vi "Main - E700 Example.vi"() -> ()   [LabVIEW 2020]
uses:
  <vilib>/NI/Modbus Library/API/Master/Modbus Master.lvclass
  C:/Program Files (x86)/National Instruments/LabVIEW 2020/vi.lib/NI/Modbus Library/API/Modbus API.lvclass
  <vilib>/NI/Modbus Library/API/Modbus API.lvclass/Modbus API.ctl
  <vilib>/NI/Modbus Library/Transmission Data Unit/Transmission Data Unit.lvclass/Transmission Data Unit.ctl
  <vilib>/NI/Modbus Library/Transmission Data Unit/Write Unit ID.vi
  <vilib>/NI/Modbus Library/API/Read Transmission Data Unit.vi
  <vilib>/NI/Modbus Library/API/Write Transmission Data Unit.vi
  <vilib>/NI/Modbus Library/API/Wrapper/Create Serial Master.vi
  <vilib>/NI/Modbus Library/API/Wrapper/API Main.lvlib
panel:
  in  "Manual Vert Control 2":bool
  in  "Vertical Direction Switch 2":bool caption="Vertical Direction Switch"
  in  "Vertical Frequencey Setting (Hz) - Manual 2":dbl caption="Vertical Frequencey Setting (Hz)" min=0.0 max=60.0 step=1.0
  in  "Rotational Frequencey Setting (Hz) - Manual 2":dbl caption="Rotational Frequencey Setting (Hz)" min=0.0 max=60.0 step=1.0
  out "Tension":bool
  out "Grease":bool
  out "D-Shape":bool
  in  "Reset Tension":bool
  in  "Reset Grease":bool
  in  "Reset D Shape":bool
  in  "Full Automated Sequence":bool
  in  "Run Full Automated Sequence":string="Sequence 3\nSequence 4\nSequence 5\nSequence 6\nSequence 7\nSequence 8\nSequence 9\nSequence 10\nSequence 11\nSequence 12"
  out "Status":string
  in  "Manual Rotational Control":bool
  in  "Rotational Frequencey Setting (Hz) - Manual 1":dbl caption="Rotational Frequencey Setting (Hz)" min=0.0 max=60.0 step=1.0
  in  "Manual Vert Control":bool
  in  "Vertical Direction Switch":bool
  in  "Vertical Frequencey Setting (Hz) - Manual 1":dbl caption="Vertical Frequencey Setting (Hz)" min=0.0 max=60.0 step=1.0
  in  "Tab Control":T1(tab)
  in  "Seq 5 Direction Switch":bool
  in  "Seq5":bool
  in  "Time (mS) - Seq 5":u32=11400 caption="Time (mS)" max=60 step=1
  in  "Rotational Frequencey Setting (Hz) - Seq 5":dbl=9.4 caption="Rotational Frequencey Setting (Hz)" min=0.0 max=60.0 step=1.0
  in  "Vertical Frequencey Setting (Hz) - Seq 5":dbl caption="Vertical Frequencey Setting (Hz)" min=0.0 max=60.0 step=1.0
  in  "Seq 4 Direction Switch":bool
  in  "Seq4":bool
  in  "Time (mS) - Seq 4":u32=5600 caption="Time (mS)" max=60 step=1
  in  "Rotational Frequencey Setting (Hz) - Seq 4":dbl caption="Rotational Frequencey Setting (Hz)" min=0.0 max=60.0 step=1.0
  in  "Vertical Frequencey Setting (Hz) - Seq 4":dbl=30.0 caption="Vertical Frequencey Setting (Hz)" min=0.0 max=60.0 step=1.0
  in  "Seq 3 Direction Switch":bool
  in  "Seq3":bool
  in  "Time (mS) - Seq 3":u32=45050 caption="Time (mS)" max=60 step=1
  in  "Rotational Frequencey Setting (Hz) - Seq 3":dbl=9.4 caption="Rotational Frequencey Setting (Hz)" min=0.0 max=60.0 step=1.0
  in  "Vertical Frequencey Setting (Hz) - Seq 3":dbl=6.9 caption="Vertical Frequencey Setting (Hz)" min=0.0 max=60.0 step=1.0
  in  "Seq 2 Direction Switch":bool
  in  "Seq2":bool
  in  "Time (mS) - Seq 2":u32=6500 caption="Time (mS)" max=60 step=1
  in  "Rotational Frequencey Setting (Hz) - Seq 2":dbl=9.4 caption="Rotational Frequencey Setting (Hz)" min=0.0 max=60.0 step=1.0
  in  "Vertical Frequencey Setting (Hz) - Seq 2":dbl=6.9 caption="Vertical Frequencey Setting (Hz)" min=0.0 max=60.0 step=1.0
  in  "COM Port":refnum<visa-resource-name>
  in  "Seq 0 Direction Switch":bool
  in  "Seq0":bool
  in  "Time (mS) - Seq 0":u32=1500 caption="Time (mS)" max=60 step=1
  in  "Rotational Frequencey Setting (Hz) - Seq 0":dbl=9.4 caption="Rotational Frequencey Setting (Hz)" min=0.0 max=60.0 step=1.0
  in  "Vertical Frequencey Setting (Hz) - Seq 0":dbl caption="Vertical Frequencey Setting (Hz)" min=0.0 max=60.0 step=1.0
  in  "Seq 1 Direction Switch":bool
  in  "Seq1":bool
  in  "Time (mS) - Seq 1":u32=4000 caption="Time (mS)" max=60 step=1
  in  "Rotational Frequencey Setting (Hz) - Seq 1":dbl=9.4 caption="Rotational Frequencey Setting (Hz)" min=0.0 max=60.0 step=1.0
  in  "Vertical Frequencey Setting (Hz) - Seq 1":dbl=6.9 caption="Vertical Frequencey Setting (Hz)" min=0.0 max=60.0 step=1.0
  in  "Seq 6 Direction Switch":bool
  in  "Seq6":bool
  in  "Time (mS) - Seq 6":u32=60040 caption="Time (mS)" max=60 step=1
  in  "Rotational Frequencey Setting (Hz) - Seq 6":dbl=9.4 caption="Rotational Frequencey Setting (Hz)" min=0.0 max=60.0 step=1.0
  in  "Vertical Frequencey Setting (Hz) - Seq 6":dbl=5.4 caption="Vertical Frequencey Setting (Hz)" min=0.0 max=60.0 step=1.0
  in  "Seq 11 Direction Switch":bool
  in  "Seq11":bool
  in  "Time (mS) - Seq 11":u32=7600 caption="Time (mS)" max=60 step=1
  in  "Rotational Frequencey Setting (Hz) - Seq 11":dbl caption="Rotational Frequencey Setting (Hz)" min=0.0 max=60.0 step=1.0
  in  "Vertical Frequencey Setting (Hz) - Seq 11":dbl=30.0 caption="Vertical Frequencey Setting (Hz)" min=0.0 max=60.0 step=1.0
  in  "Seq 10 Direction Switch":bool
  in  "Seq10":bool
  in  "Time (mS) - Seq 10":u32=134850 caption="Time (mS)" max=60 step=1
  in  "Rotational Frequencey Setting (Hz) - Seq 10":dbl=9.4 caption="Rotational Frequencey Setting (Hz)" min=0.0 max=60.0 step=1.0
  in  "Vertical Frequencey Setting (Hz) - Seq 10":dbl=2.75 caption="Vertical Frequencey Setting (Hz)" min=0.0 max=60.0 step=1.0
  in  "Seq 9 Direction Switch":bool
  in  "Seq9":bool
  in  "Time (mS) - Seq 9":u32=45050 caption="Time (mS)" max=60 step=1
  in  "Rotational Frequencey Setting (Hz) - Seq 9":dbl=9.4 caption="Rotational Frequencey Setting (Hz)" min=0.0 max=60.0 step=1.0
  in  "Vertical Frequencey Setting (Hz) - Seq 9":dbl=5.4 caption="Vertical Frequencey Setting (Hz)" min=0.0 max=60.0 step=1.0
  in  "Seq 8 Direction Switch":bool
  in  "Seq8":bool
  in  "Time (mS) - Seq 8":u32=11400 caption="Time (mS)" max=60 step=1
  in  "Rotational Frequencey Setting (Hz) - Seq 8":dbl=9.4 caption="Rotational Frequencey Setting (Hz)" min=0.0 max=60.0 step=1.0
  in  "Vertical Frequencey Setting (Hz) - Seq 8":dbl caption="Vertical Frequencey Setting (Hz)" min=0.0 max=60.0 step=1.0
  in  "Seq 7 Direction Switch":bool
  in  "Seq7":bool
  in  "Time (mS) - Seq 7":u32=10900 caption="Time (mS)" max=60 step=1
  in  "Rotational Frequencey Setting (Hz) - Seq 7":dbl caption="Rotational Frequencey Setting (Hz)" min=0.0 max=60.0 step=1.0
  in  "Vertical Frequencey Setting (Hz) - Seq 7":dbl=30.0 caption="Vertical Frequencey Setting (Hz)" min=0.0 max=60.0 step=1.0
  in  "Seq 12 Direction Switch":bool
  in  "Seq12":bool
  in  "Time (mS) - Seq 12":u32=17034 caption="Time (mS)" max=60 step=1
  in  "Rotational Frequencey Setting (Hz) - Seq 12":dbl=9.4 caption="Rotational Frequencey Setting (Hz)" min=0.0 max=60.0 step=1.0
  in  "Vertical Frequencey Setting (Hz) - Seq 12":dbl=4.6 caption="Vertical Frequencey Setting (Hz)" min=0.0 max=60.0 step=1.0
  in  "Seq 15 Direction Switch":bool
  in  "Seq15":bool
  in  "Time (mS) - Seq 15":u32=13000 caption="Time (mS)" max=60 step=1
  in  "Rotational Frequencey Setting (Hz) - Seq 15":dbl=9.4 caption="Rotational Frequencey Setting (Hz)" min=0.0 max=60.0 step=1.0
  in  "Vertical Frequencey Setting (Hz) - Seq 15":dbl=4.6 caption="Vertical Frequencey Setting (Hz)" min=0.0 max=60.0 step=1.0
  in  "Seq 14 Direction Switch":bool
  in  "Seq14":bool
  in  "Time (mS) - Seq 14":u32=11060 caption="Time (mS)" max=60 step=1
  in  "Rotational Frequencey Setting (Hz) - Seq 14":dbl=9.4 caption="Rotational Frequencey Setting (Hz)" min=0.0 max=60.0 step=1.0
  in  "Vertical Frequencey Setting (Hz) - Seq 14":dbl=4.6 caption="Vertical Frequencey Setting (Hz)" min=0.0 max=60.0 step=1.0
  in  "Seq 13 Direction Switch":bool
  in  "Seq13":bool
  in  "Time (mS) - Seq 13":u32=4209 caption="Time (mS)" max=60 step=1
  in  "Rotational Frequencey Setting (Hz) - Seq 13":dbl=9.4 caption="Rotational Frequencey Setting (Hz)" min=0.0 max=60.0 step=1.0
  in  "Vertical Frequencey Setting (Hz) - Seq 13":dbl=4.6 caption="Vertical Frequencey Setting (Hz)" min=0.0 max=60.0 step=1.0
  out "Rotational Frequency Output":dbl
  out "Vertical Frequency Output":dbl
  in  "OK":bool
  # "Manual Control - Rotational"
  # "Manual Control-Vertical"
  # "Combination Control-Rotational and Vertical"
  # "Sequence 2 - Install Clamp at END and Turn Tension ON at END"
  # "Sequence 3 - Three Revolutions"
  # "Sequence 4 - Vertical Drop"
  # "Sequence 5 - 3/4 Turn Offset"
  # "Sequence 6 - Four Revolutions"
  # "Sequence 0 - Tension Offset and Start D at END"
  # "Sequence 1 - Start Grease at END"
  # "Sequence 7 - Vertical Drop"
  # "Sequence 8 - 3/4 Turn Offset"
  # "Sequence 9 - Three Revolutions"
  # "Sequence 10 - Nine Revolutions"
  # "Sequence 11 - Vertical Drop"
  # "Sequence 12 - One Revolution + 45 Degrees - Turn D off at END"
  # "Sequence 13 - 100 Degree Revolution, Turn Grease off at END"
  # "Sequence 14 - Finish Revolution and Install Clamp and Turn Tension OFF at END"
  # "Sequence 15 - Create Tail"
  # "Channel 79 needs to be set from 3 to 2 - Power must be cycled."
  # "21.5\" Diameter Tank:\nSequence 0 (mS): 1500\nSequence 1 (mS): 4000\nSequence 2 (mS): 6500\nSequence 3 (mS): 45000\nSequence 4 (mS): 5600\nSequence 5 (mS): 11500\nSequence 6 (mS): 50000\nSequence 7 (mS): 10900\nSequence 8 (mS): 10500\nSequence 9 (mS): 33750\nSequence 10 (mS): 137000\nSequence 11 (mS): 7600\nSequence 12 (mS): 16500\nSequence 13 (mS): 3000 \nSequence 14 (mS): 10000\nSequence 15 (mS): 13000"
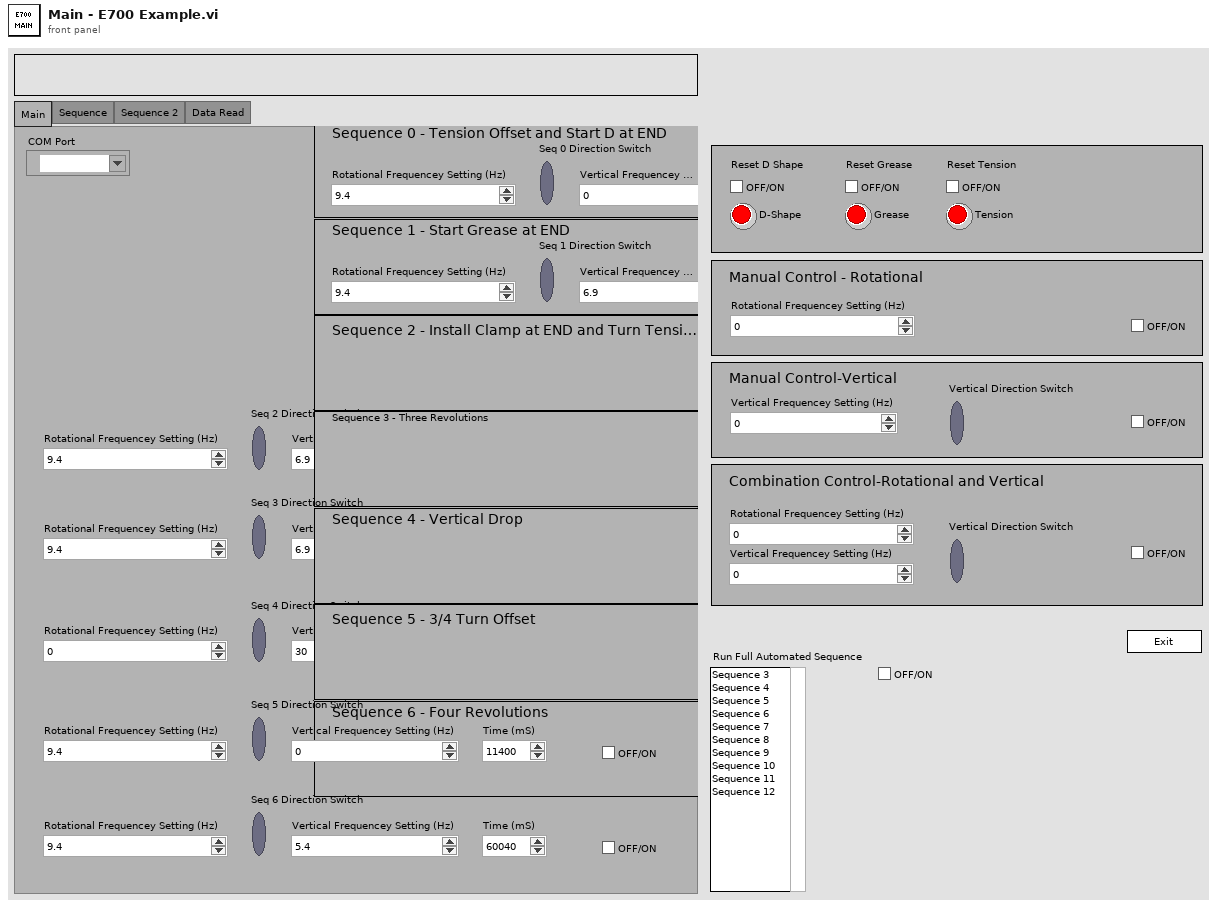
[diagram p1: front panel]
types:
  T1 = enum32{"Main", "Sequence", "Sequence 2", "Data Read"}
  T2 = enum32{"Invalid", "Standard", "Closed", "Hidden", "Minimized", "Maximized"}
  T3 = enum32{"invalid app kind", "Development System", "Run Time System", "Student Edition", "Embedded LabVIEW", "Evaluation", "Custom"}
  T4 = cluster{"Core":cluster{"Current VI Reference":refnum<vi>, "Close Panel on Exit?":bool}, "COM Port":refnum<visa-resource-name>, "Rotation Instance":refnum<class "Modbus Master.lvclass">, "Tension":bool, "D Shape":bool, "Grease":bool}
  T5 = cluster{"Current VI Reference":refnum<vi>, "Close Panel on Exit?":bool}
  T6 = cluster{"register values[0]":u16, "register values[1]":u16, "register values[2]":u16, "register values[3]":u16, "register values[4]":u16, "register values[5]":u16, "register values[6]":u16, "register values[7]":u16, "register values[8]":u16}
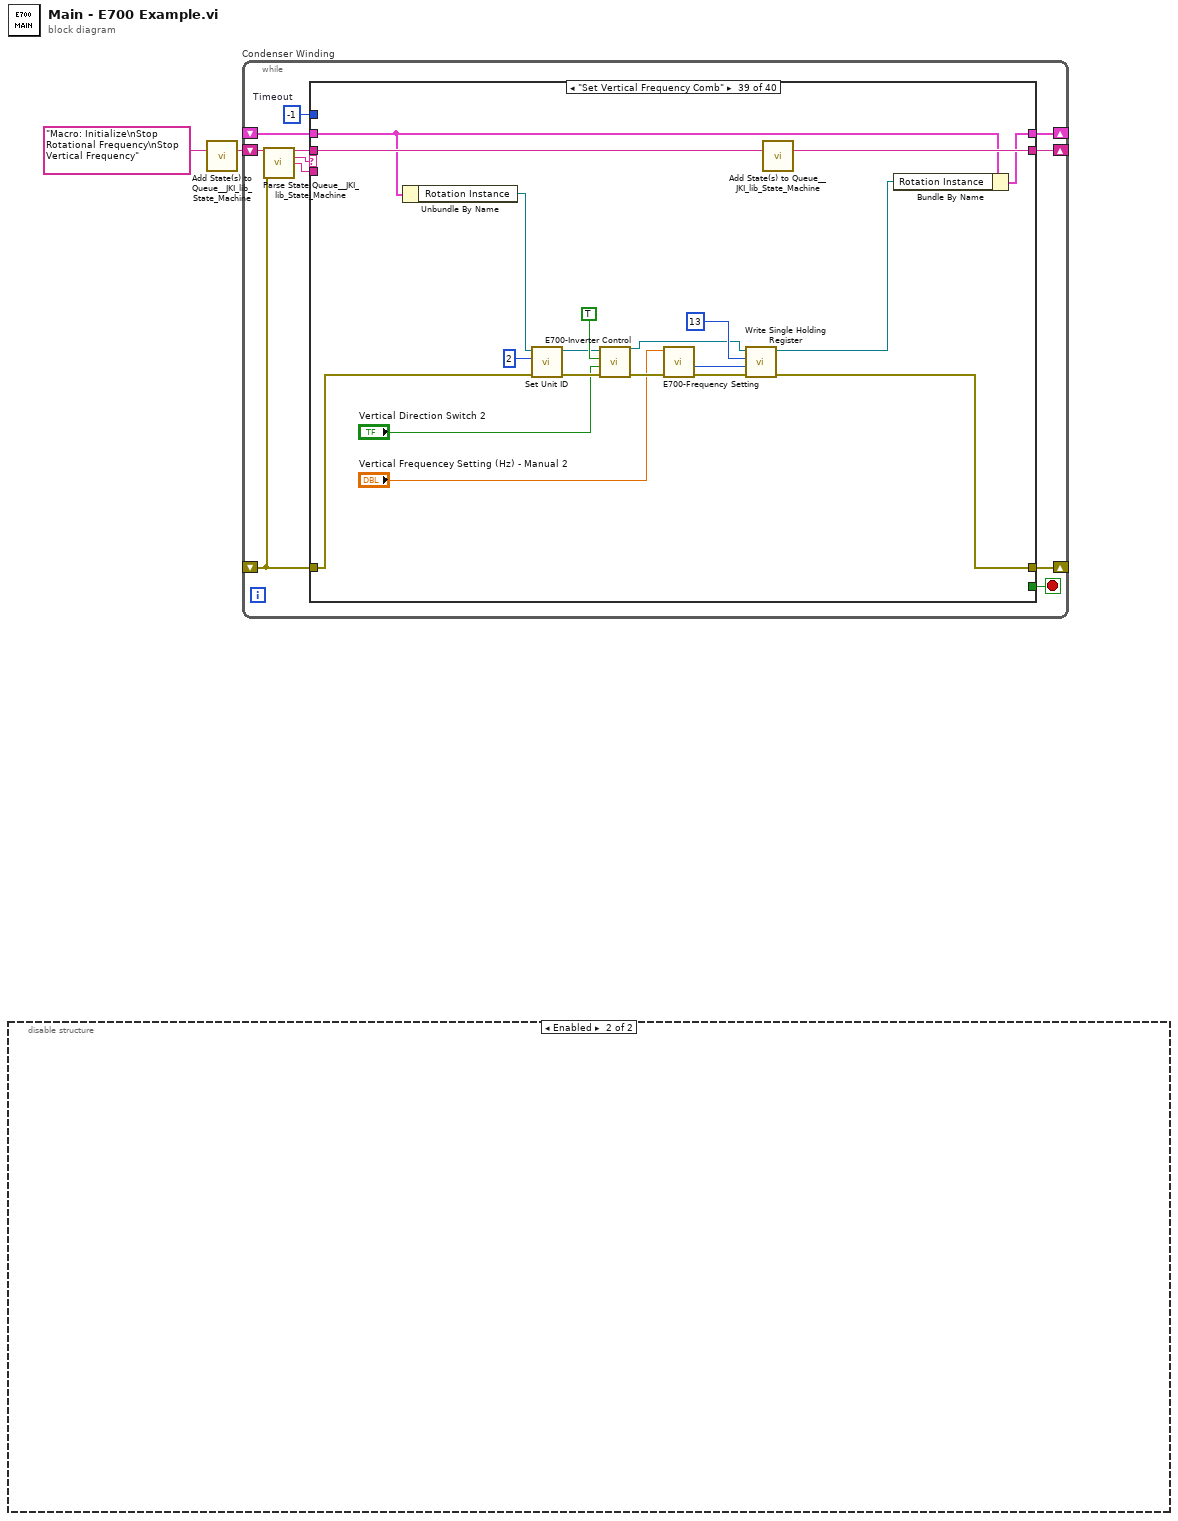
[diagram p0: block diagram]
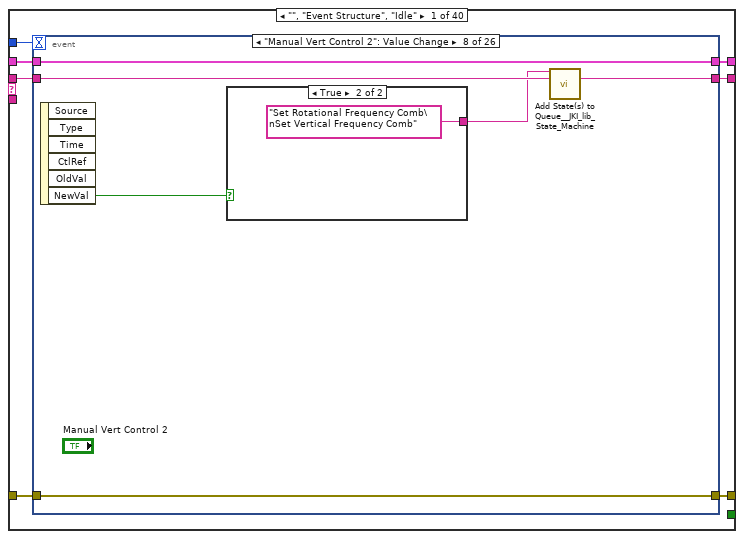
[diagram p2: hidden frame]
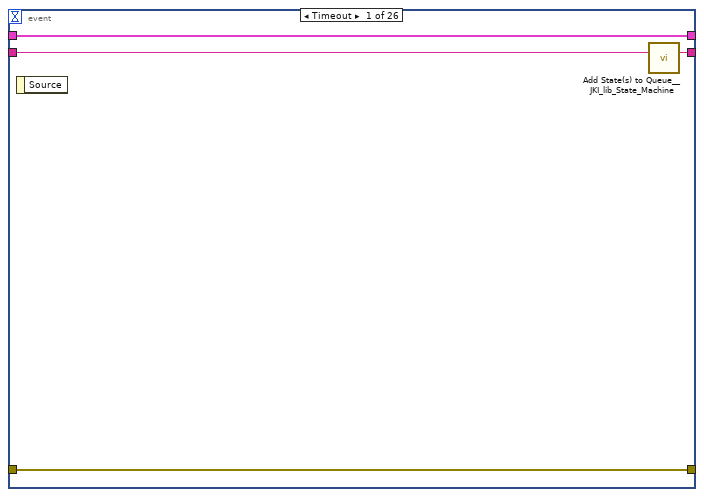
[diagram p3: hidden frame]
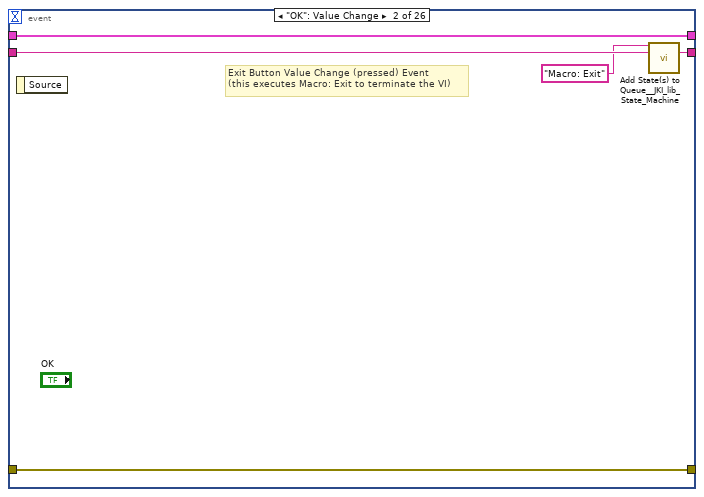
[diagram p4: hidden frame]
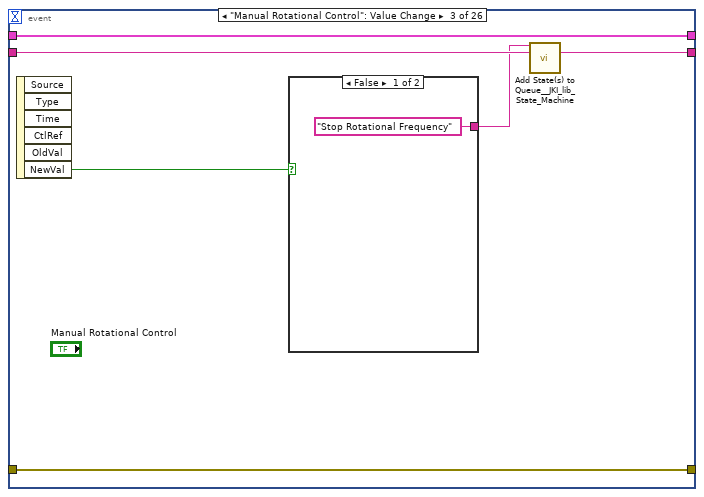
[diagram p5: hidden frame]
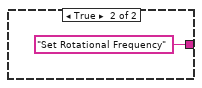
[diagram p6: hidden frame]
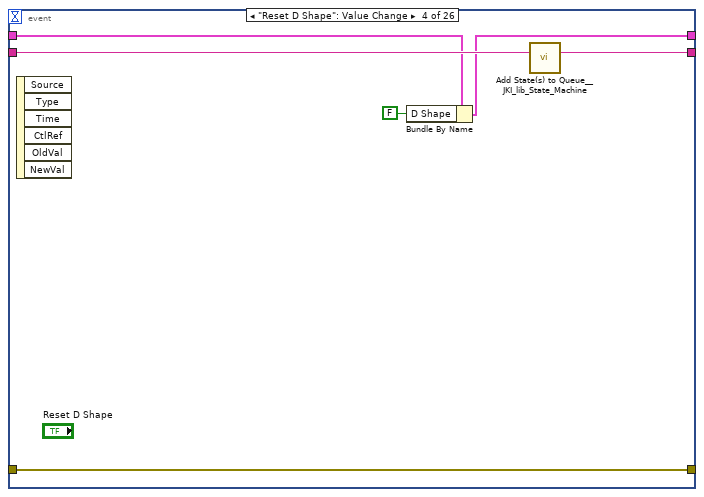
[diagram p7: hidden frame]
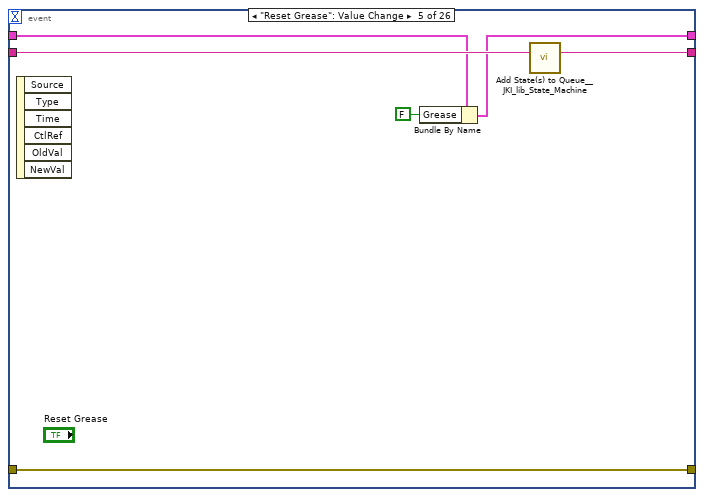
[diagram p8: hidden frame]
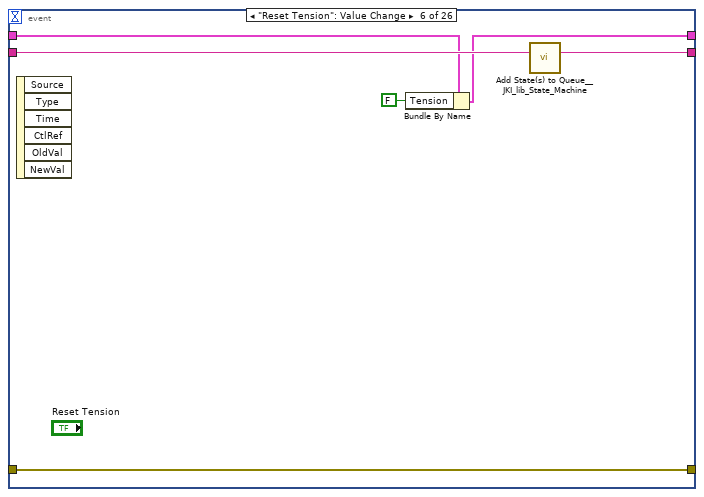
[diagram p9: hidden frame]
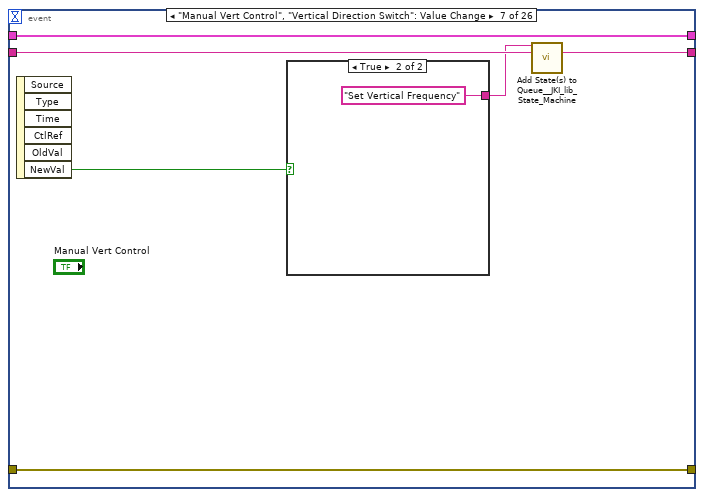
[diagram p10: hidden frame]
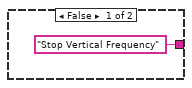
[diagram p11: hidden frame]
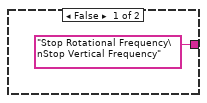
[diagram p12: hidden frame]
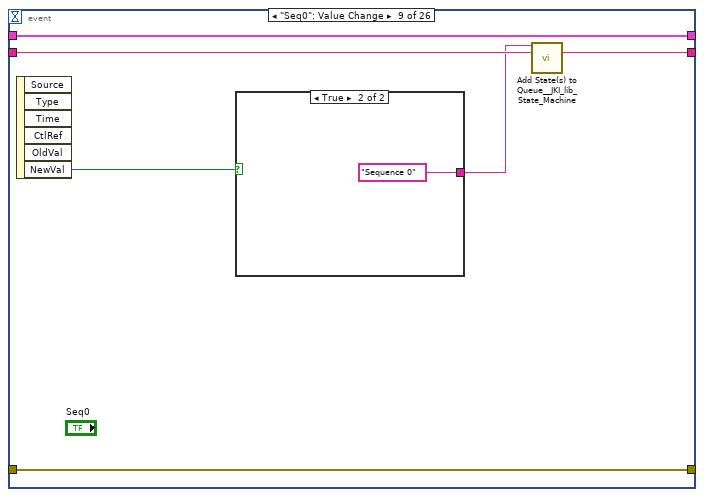
[diagram p13: hidden frame]
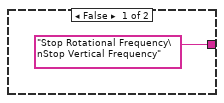
[diagram p14: hidden frame]
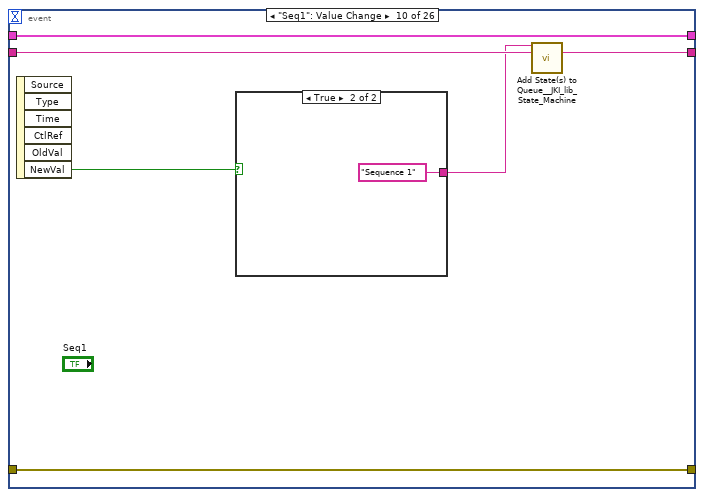
[diagram p15: hidden frame]
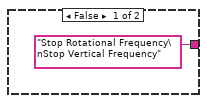
[diagram p16: hidden frame]
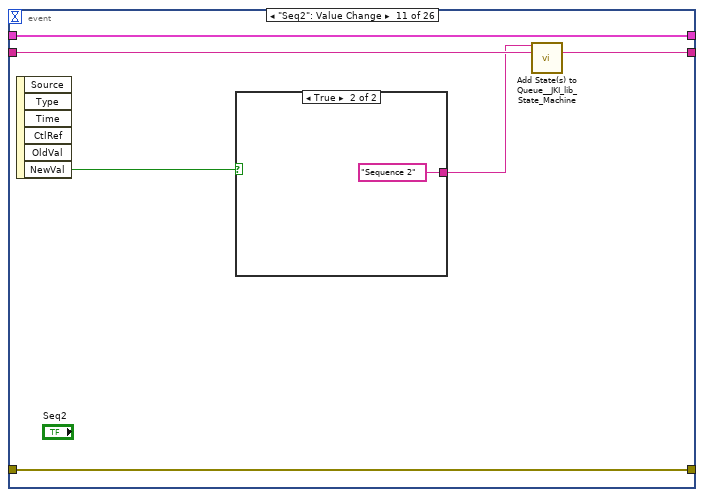
[diagram p17: hidden frame]
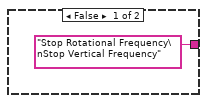
[diagram p18: hidden frame]
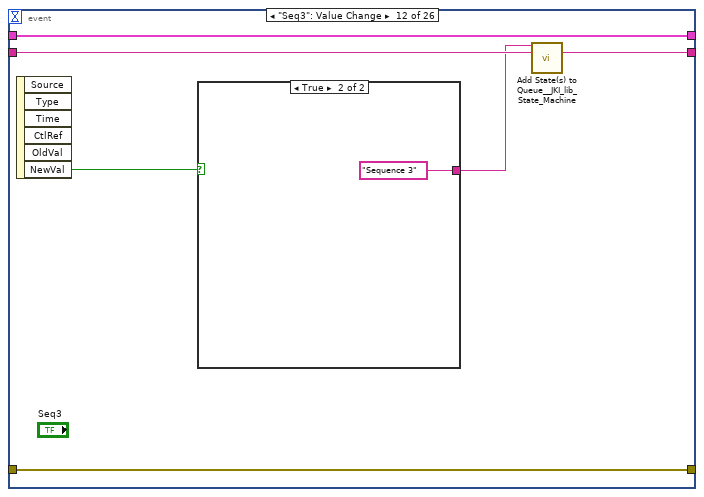
[diagram p19: hidden frame]
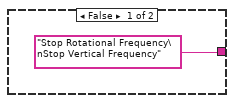
[diagram p20: hidden frame]
diagram:
  n1 = disable-structure shown="Enabled" {
    frame Disabled {
    }
    frame Enabled {
    }
  }
  n2 = call <vilib>:"Add State(s) to Queue__JKI_lib_State_Machine.vi"("State(s) in (\"\")"="Macro: Initialize\nStop Rotational Frequency\nStop Vertical Frequency") -> ("States Out"=w2:string)  [unwired: 14 in]
  n3 = while "Condenser Winding" {
    shift-right: [w6] -> _
    shift-left: _ -> [w5]
    shift-right: [w9] -> _
    shift-left: _ -> [w3]
    shift-right: [w8] -> _
    shift-left: w2 -> [w10]
    stop <- w7 stop-if-true
    w4 = -1  # Timeout
    n4 = call <vilib>:"Parse State Queue__JKI_lib_State_Machine.vi"("State Queue"=w10, "Error In (no error)"=w3) -> ("Remaining States"=w12:string, "Current State"=w13:string, "Arguments"=w11:string)  [unwired: 11 in]
    n5 = case shown="\"Set Vertical Frequency Comb\"" w13 {
      selector: w13 -> [_ _ w218 _ _ _ _ _ _ _ _ _ _ _ _ _ _ _ _ _ _ _ _ _ _ _ _ _ _ _ _ _ _ _ _ _ _ _ _ _]
      tunnel: w12 -> [w20 w217 w222 w241 w247 w254 w258 w268 w274 w278 w292 w298 w309 w378 w383 w393 w397 w410 w427 w444 w459 w472 w489 w504 w517 w534 w549 w560 w573 w592 w613 w630 w645 w650 w687 w702 w717 w736 w755 w767]
      tunnel: w11 -> [_ _ _ _ _ _ _ _ _ _ _ w293 w303 _ _ _ _ _ _ _ _ _ _ _ _ _ _ _ _ _ _ _ _ _ _ _ _ _ _ _]
      tunnel: w5 -> [w18 w214 w220 w234 w244 w251 w255 _ w269 w275 w284 w296 w305 w375 w380 w390 w394 w399 w415 w432 w457 w464 w481 w502 w509 w526 w547 w558 w565 w581 w603 w619 w643 w648 w681 w696 w711 w730 w749 w764]
      tunnel: [w17 w215 w224 w238 errorcluster {"status"=FALSE, "code"=0, "source"=""} ("error out") w250 w256 w265 w270 w276 w280 w294 w306 w376 w381 w391 w395 w400 w417 w434 w455 w461 w477 w496 w505 w522 w544 w555 w561 w583 w601 w618 w640 w646 w682 w697 w712 w718 w739 w763] -> w9
      tunnel: w3 -> [w16 w215 w223 w238 w243 w248 w256 w265 w271 w276 w286 w295 w307 w376 w381 w391 w395 w408 w425 w441 w456 w463 w479 w501 w507 w523 w546 w557 w563 w579 w611 w628 w642 w647 w683 w698 w713 w722 w743 w757]
      tunnel: [w19 w216 w221 w240 w246 w253 w257 w267 w273 w277 w291 w297 w308 w377 w382 w392 w396 w409 w426 w443 w458 w471 w488 w503 w516 w533 w548 w559 w572 w591 w612 w629 w644 w649 w686 w701 w716 w735 w754 w766] -> w8
      tunnel: [_ _ _ _ _ TRUE _ _ _ _ _ _ _ _ _ _ _ _ _ _ _ _ _ _ _ _ _ _ _ _ _ _ _ _ _ _ _ _ _ _] -> w7
      tunnel: [w15 w214 w220 w239 w244 w251 w255 w266 w269 w275 w283 w296 w305 w375 w380 w390 w394 w398 w416 w433 w457 w460 w478 w502 w508 w525 w547 w558 w564 w582 w604 w620 w643 w648 w680 w695 w710 w731 w750 w765] -> w6
      tunnel: w4 -> [w14 _ _ _ _ _ _ _ _ _ _ _ _ _ _ _ _ _ _ _ _ _ _ _ _ _ _ _ _ _ _ _ _ _ _ _ _ _ _ _]
      frame "", "Event Structure", "Idle" {
        n6 = event shown="[7] \"Manual Vert Control 2\": Value Change" {
          selector: _ -> [_ _ _ _ _ _ _ _ _ _ _ _ _ _ _ _ _ _ _ _ _ _ _ _ _ _]
          dyn-events: _ -> [_ _ _ _ _ _ _ _ _ _ _ _ _ _ _ _ _ _ _ _ _ _ _ _ _ _]
          timeout: w14 -> [_ _ _ _ _ _ _ _ _ _ _ _ _ _ _ _ _ _ _ _ _ _ _ _ _ _]
          tunnel: w20 -> [w24 w29 w34 w43 w49 w55 w58 w67 w74 w82 w90 w98 w106 w114 w122 w130 w138 w146 w154 w162 w170 w178 w186 w194 w202 w213]
          tunnel: [w23 w28 w33 w42 w48 w54 w59 w66 w75 w83 w91 w99 w107 w115 w123 w131 w139 w147 w155 w163 w171 w179 w187 w195 w203 w212] -> w19
          tunnel: w18 -> [w21 w26 w35 w40 w46 w52 w61 w69 w77 w85 w93 w101 w109 w117 w125 w133 w141 w149 w157 w165 w173 w181 w189 w197 w205 w210]
          tunnel: [w22 w27 w31 w41 w47 w53 w60 w68 w76 w84 w92 w100 w108 w116 w124 w132 w140 w148 w156 w164 w172 w180 w188 w196 w204 w211] -> w17
          tunnel: w16 -> [w22 w27 w31 w41 w47 w53 w60 w68 w76 w84 w92 w100 w108 w116 w124 w132 w140 w148 w156 w164 w172 w180 w188 w196 w204 w211]
          tunnel: [w21 w26 w35 w39 w45 w51 w61 w69 w77 w85 w93 w101 w109 w117 w125 w133 w141 w149 w157 w165 w173 w181 w189 w197 w205 w210] -> w15
          event Timeout {
            n7 = event-data() -> ()  [unwired: 1 in, 1 out]
            n8 = call <vilib>:"Add State(s) to Queue__JKI_lib_State_Machine.vi"("State(s) in (\"\")"=w24) -> ("States Out"=w23:string)  [unwired: 14 in]
          }
          event "OK": Value Change {
            # "Exit Button Value Change (pressed) Event\n(this executes Macro: Exit to terminate the VI)"
            n9 = event-data() -> ()  [unwired: 1 in, 1 out]
            n10 = call <vilib>:"Add State(s) to Queue__JKI_lib_State_Machine.vi"("State(s) in Front (\"\")"="Macro: Exit", "State(s) in (\"\")"=w29) -> ("States Out"=w28:string)  [unwired: 13 in]
          }
          event "Manual Rotational Control": Value Change {
            n11 = event-data() -> ("NewVal"=w30:bool)  [unwired: 1 in, 5 out]
            n12 = case shown="False" w30 {
              tunnel: ["Stop Rotational Frequency" ("State(s) in Front (\"\")") "Set Rotational Frequency" ("State(s) in Front (\"\")")] -> w32
              frame False {
              }
              frame True {
              }
            }
            n13 = call <vilib>:"Add State(s) to Queue__JKI_lib_State_Machine.vi"("State(s) in Front (\"\")"=w32, "State(s) in (\"\")"=w34) -> ("States Out"=w33:string)  [unwired: 13 in]
          }
          event "Reset D Shape": Value Change {
            n14 = event-data() -> ()  [unwired: 1 in, 6 out]
            n15 = Bundle By Name(cluster=w40, "D Shape"=FALSE) -> (w39:T4)
            n16 = call <vilib>:"Add State(s) to Queue__JKI_lib_State_Machine.vi"("State(s) in (\"\")"=w43) -> ("States Out"=w42:string)  [unwired: 14 in]
          }
          event "Reset Grease": Value Change {
            n17 = event-data() -> ()  [unwired: 1 in, 6 out]
            n18 = Bundle By Name(cluster=w46, "Grease"=FALSE) -> (w45:T4)
            n19 = call <vilib>:"Add State(s) to Queue__JKI_lib_State_Machine.vi"("State(s) in (\"\")"=w49) -> ("States Out"=w48:string)  [unwired: 14 in]
          }
          event "Reset Tension": Value Change {
            n20 = event-data() -> ()  [unwired: 1 in, 6 out]
            n21 = Bundle By Name(cluster=w52, "Tension"=FALSE) -> (w51:T4)
            n22 = call <vilib>:"Add State(s) to Queue__JKI_lib_State_Machine.vi"("State(s) in (\"\")"=w55) -> ("States Out"=w54:string)  [unwired: 14 in]
          }
          event "Manual Vert Control", "Vertical Direction Switch": Value Change {
            n23 = event-data() -> ("NewVal"=w56:bool)  [unwired: 1 in, 5 out]
            n24 = case shown="True" w56 {
              tunnel: ["Stop Vertical Frequency" ("State(s) in Front (\"\")") "Set Vertical Frequency" ("State(s) in Front (\"\")")] -> w57
              frame False {
              }
              frame True {
              }
            }
            n25 = call <vilib>:"Add State(s) to Queue__JKI_lib_State_Machine.vi"("State(s) in Front (\"\")"=w57, "State(s) in (\"\")"=w58) -> ("States Out"=w59:string)  [unwired: 13 in]
          }
          event "Manual Vert Control 2": Value Change {
            n26 = event-data() -> ("NewVal"=w65:bool)  [unwired: 1 in, 5 out]
            n27 = case shown="True" w65 {
              tunnel: ["Stop Rotational Frequency\nStop Vertical Frequency" ("State(s) in Front (\"\")") "Set Rotational Frequency Comb\nSet Vertical Frequency Comb" ("State(s) in Front (\"\")")] -> w64
              frame False {
              }
              frame True {
              }
            }
            n28 = call <vilib>:"Add State(s) to Queue__JKI_lib_State_Machine.vi"("State(s) in Front (\"\")"=w64, "State(s) in (\"\")"=w67) -> ("States Out"=w66:string)  [unwired: 13 in]
          }
          event "Seq0": Value Change {
            n29 = event-data() -> ("NewVal"=w72:bool)  [unwired: 1 in, 5 out]
            n30 = case shown="True" w72 {
              tunnel: ["Stop Rotational Frequency\nStop Vertical Frequency" ("State(s) in Front (\"\")") "Sequence 0" ("State(s) in Front (\"\")")] -> w73
              frame False {
              }
              frame True {
              }
            }
            n31 = call <vilib>:"Add State(s) to Queue__JKI_lib_State_Machine.vi"("State(s) in Front (\"\")"=w73, "State(s) in (\"\")"=w74) -> ("States Out"=w75:string)  [unwired: 13 in]
          }
          event "Seq1": Value Change {
            n32 = event-data() -> ("NewVal"=w80:bool)  [unwired: 1 in, 5 out]
            n33 = case shown="True" w80 {
              tunnel: ["Stop Rotational Frequency\nStop Vertical Frequency" ("State(s) in Front (\"\")") "Sequence 1" ("State(s) in Front (\"\")")] -> w81
              frame False {
              }
              frame True {
              }
            }
            n34 = call <vilib>:"Add State(s) to Queue__JKI_lib_State_Machine.vi"("State(s) in Front (\"\")"=w81, "State(s) in (\"\")"=w82) -> ("States Out"=w83:string)  [unwired: 13 in]
          }
          event "Seq2": Value Change {
            n35 = event-data() -> ("NewVal"=w88:bool)  [unwired: 1 in, 5 out]
            n36 = case shown="True" w88 {
              tunnel: ["Stop Rotational Frequency\nStop Vertical Frequency" ("State(s) in Front (\"\")") "Sequence 2" ("State(s) in Front (\"\")")] -> w89
              frame False {
              }
              frame True {
              }
            }
            n37 = call <vilib>:"Add State(s) to Queue__JKI_lib_State_Machine.vi"("State(s) in Front (\"\")"=w89, "State(s) in (\"\")"=w90) -> ("States Out"=w91:string)  [unwired: 13 in]
          }
          event "Seq3": Value Change {
            n38 = event-data() -> ("NewVal"=w96:bool)  [unwired: 1 in, 5 out]
            n39 = case shown="True" w96 {
              tunnel: ["Stop Rotational Frequency\nStop Vertical Frequency" ("State(s) in Front (\"\")") "Sequence 3" ("State(s) in Front (\"\")")] -> w97
              frame False {
              }
              frame True {
              }
            }
            n40 = call <vilib>:"Add State(s) to Queue__JKI_lib_State_Machine.vi"("State(s) in Front (\"\")"=w97, "State(s) in (\"\")"=w98) -> ("States Out"=w99:string)  [unwired: 13 in]
          }
          event "Seq4": Value Change {
            n41 = event-data() -> ("NewVal"=w104:bool)  [unwired: 1 in, 5 out]
            n42 = case shown="True" w104 {
              tunnel: ["Stop Rotational Frequency\nStop Vertical Frequency" ("State(s) in Front (\"\")") "Sequence 4" ("State(s) in Front (\"\")")] -> w105
              frame False {
              }
              frame True {
              }
            }
            n43 = call <vilib>:"Add State(s) to Queue__JKI_lib_State_Machine.vi"("State(s) in Front (\"\")"=w105, "State(s) in (\"\")"=w106) -> ("States Out"=w107:string)  [unwired: 13 in]
          }
          event "Seq5": Value Change {
            n44 = event-data() -> ("NewVal"=w112:bool)  [unwired: 1 in, 5 out]
            n45 = case shown="True" w112 {
              tunnel: ["Stop Rotational Frequency\nStop Vertical Frequency" ("State(s) in Front (\"\")") "Sequence 5" ("State(s) in Front (\"\")")] -> w113
              frame False {
              }
              frame True {
              }
            }
            n46 = call <vilib>:"Add State(s) to Queue__JKI_lib_State_Machine.vi"("State(s) in Front (\"\")"=w113, "State(s) in (\"\")"=w114) -> ("States Out"=w115:string)  [unwired: 13 in]
          }
          event "Seq6": Value Change {
            n47 = event-data() -> ("NewVal"=w120:bool)  [unwired: 1 in, 5 out]
            n48 = case shown="True" w120 {
              tunnel: ["Stop Rotational Frequency\nStop Vertical Frequency" ("State(s) in Front (\"\")") "Sequence 6" ("State(s) in Front (\"\")")] -> w121
              frame False {
              }
              frame True {
              }
            }
            n49 = call <vilib>:"Add State(s) to Queue__JKI_lib_State_Machine.vi"("State(s) in Front (\"\")"=w121, "State(s) in (\"\")"=w122) -> ("States Out"=w123:string)  [unwired: 13 in]
          }
          event "Seq7": Value Change {
            n50 = event-data() -> ("NewVal"=w128:bool)  [unwired: 1 in, 5 out]
            n51 = case shown="True" w128 {
              tunnel: ["Stop Rotational Frequency\nStop Vertical Frequency" ("State(s) in Front (\"\")") "Sequence 7" ("State(s) in Front (\"\")")] -> w129
              frame False {
              }
              frame True {
              }
            }
            n52 = call <vilib>:"Add State(s) to Queue__JKI_lib_State_Machine.vi"("State(s) in Front (\"\")"=w129, "State(s) in (\"\")"=w130) -> ("States Out"=w131:string)  [unwired: 13 in]
          }
          event "Seq8": Value Change {
            n53 = event-data() -> ("NewVal"=w136:bool)  [unwired: 1 in, 5 out]
            n54 = case shown="True" w136 {
              tunnel: ["Stop Rotational Frequency\nStop Vertical Frequency" ("State(s) in Front (\"\")") "Sequence 8" ("State(s) in Front (\"\")")] -> w137
              frame False {
              }
              frame True {
              }
            }
            n55 = call <vilib>:"Add State(s) to Queue__JKI_lib_State_Machine.vi"("State(s) in Front (\"\")"=w137, "State(s) in (\"\")"=w138) -> ("States Out"=w139:string)  [unwired: 13 in]
          }
          event "Seq9": Value Change {
            n56 = event-data() -> ("NewVal"=w144:bool)  [unwired: 1 in, 5 out]
            n57 = case shown="True" w144 {
              tunnel: ["Stop Rotational Frequency\nStop Vertical Frequency" ("State(s) in Front (\"\")") "Sequence 9" ("State(s) in Front (\"\")")] -> w145
              frame False {
              }
              frame True {
              }
            }
            n58 = call <vilib>:"Add State(s) to Queue__JKI_lib_State_Machine.vi"("State(s) in Front (\"\")"=w145, "State(s) in (\"\")"=w146) -> ("States Out"=w147:string)  [unwired: 13 in]
          }
          event "Seq10": Value Change {
            n59 = event-data() -> ("NewVal"=w152:bool)  [unwired: 1 in, 5 out]
            n60 = case shown="True" w152 {
              tunnel: ["Stop Rotational Frequency\nStop Vertical Frequency" ("State(s) in Front (\"\")") "Sequence 10" ("State(s) in Front (\"\")")] -> w153
              frame False {
              }
              frame True {
              }
            }
            n61 = call <vilib>:"Add State(s) to Queue__JKI_lib_State_Machine.vi"("State(s) in Front (\"\")"=w153, "State(s) in (\"\")"=w154) -> ("States Out"=w155:string)  [unwired: 13 in]
          }
          event "Seq11": Value Change {
            n62 = event-data() -> ("NewVal"=w160:bool)  [unwired: 1 in, 5 out]
            n63 = case shown="True" w160 {
              tunnel: ["Stop Rotational Frequency\nStop Vertical Frequency" ("State(s) in Front (\"\")") "Sequence 11" ("State(s) in Front (\"\")")] -> w161
              frame False {
              }
              frame True {
              }
            }
            n64 = call <vilib>:"Add State(s) to Queue__JKI_lib_State_Machine.vi"("State(s) in Front (\"\")"=w161, "State(s) in (\"\")"=w162) -> ("States Out"=w163:string)  [unwired: 13 in]
          }
          event "Seq12": Value Change {
            n65 = event-data() -> ("NewVal"=w168:bool)  [unwired: 1 in, 5 out]
            n66 = case shown="True" w168 {
              tunnel: ["Stop Rotational Frequency\nStop Vertical Frequency" ("State(s) in Front (\"\")") "Sequence 12" ("State(s) in Front (\"\")")] -> w169
              frame False {
              }
              frame True {
              }
            }
            n67 = call <vilib>:"Add State(s) to Queue__JKI_lib_State_Machine.vi"("State(s) in Front (\"\")"=w169, "State(s) in (\"\")"=w170) -> ("States Out"=w171:string)  [unwired: 13 in]
          }
          event "Seq13": Value Change {
            n68 = event-data() -> ("NewVal"=w176:bool)  [unwired: 1 in, 5 out]
            n69 = case shown="True" w176 {
              tunnel: ["Stop Rotational Frequency\nStop Vertical Frequency" ("State(s) in Front (\"\")") "Sequence 13" ("State(s) in Front (\"\")")] -> w177
              frame False {
              }
              frame True {
              }
            }
            n70 = call <vilib>:"Add State(s) to Queue__JKI_lib_State_Machine.vi"("State(s) in Front (\"\")"=w177, "State(s) in (\"\")"=w178) -> ("States Out"=w179:string)  [unwired: 13 in]
          }
          event "Seq14": Value Change {
            n71 = event-data() -> ("NewVal"=w184:bool)  [unwired: 1 in, 5 out]
            n72 = case shown="True" w184 {
              tunnel: ["Stop Rotational Frequency\nStop Vertical Frequency" ("State(s) in Front (\"\")") "Sequence 14" ("State(s) in Front (\"\")")] -> w185
              frame False {
              }
              frame True {
              }
            }
            n73 = call <vilib>:"Add State(s) to Queue__JKI_lib_State_Machine.vi"("State(s) in Front (\"\")"=w185, "State(s) in (\"\")"=w186) -> ("States Out"=w187:string)  [unwired: 13 in]
          }
          event "Seq15": Value Change {
            n74 = event-data() -> ("NewVal"=w192:bool)  [unwired: 1 in, 5 out]
            n75 = case shown="True" w192 {
              tunnel: ["Stop Rotational Frequency\nStop Vertical Frequency" ("State(s) in Front (\"\")") "Sequence 15" ("State(s) in Front (\"\")")] -> w193
              frame False {
              }
              frame True {
              }
            }
            n76 = call <vilib>:"Add State(s) to Queue__JKI_lib_State_Machine.vi"("State(s) in Front (\"\")"=w193, "State(s) in (\"\")"=w194) -> ("States Out"=w195:string)  [unwired: 13 in]
          }
          event "Full Automated Sequence": Value Change {
            n77 = event-data() -> ("NewVal"=w200:bool)  [unwired: 1 in, 5 out]
            n78 = case shown="False" w200 {
              tunnel: ["Stop Rotational Frequency\nStop Vertical Frequency" ("State(s) in Front (\"\")") "Run Full Automated Sequence"] -> w201
              frame False {
              }
              frame True {
              }
            }
            n79 = call <vilib>:"Add State(s) to Queue__JKI_lib_State_Machine.vi"("State(s) in Front (\"\")"=w201, "State(s) in (\"\")"=w202) -> ("States Out"=w203:string)  [unwired: 13 in]
          }
          event Panel Close? {
            # "Discard the event because we'll close the front panel ourselves in Macro: Exit"
            # "Close Panel button (pressed) Event\n(this executes Macro: Exit to terminate the VI)"
            n80 = event-data() -> ()  [unwired: 1 in, 1 out]
            n81 = event-data("Discard?"=TRUE) -> ()  [unwired: 1 in, 1 out]
            n82 = call <vilib>:"Add State(s) to Queue__JKI_lib_State_Machine.vi"("State(s) in Front (\"\")"="Macro: Exit", "State(s) in (\"\")"=w213) -> ("States Out"=w212:string)  [unwired: 13 in]
          }
        }
      }
      frame "---------- Core ----------" {
        # "Do not put any code in this frame.\n(it is a separator no-op)"
        n83 = call <vilib>:"Add State(s) to Queue__JKI_lib_State_Machine.vi"("State(s) in (\"\")"=w217) -> ("States Out"=w216:string)  [unwired: 14 in]
      }
      frame Default {
        w227 = 42 items=["No error", "Argument error", "Memory is full", "Out of zone", "End of file", "File already open", "Generic file I/O error", "File not found", "File permission error", "Disk is full", "Duplicate path", "Too many files open", "System feature not enabled", "Resource file not found", "Cannot add resource", "Resource not found", "Image not found", "Image memory error", "Pen does not exist", "Config type invalid", "Config token not found", "Config parse error", "Config memory error", "Bad external code format", "Bad external code offset", "External code not present", "Null window", "Destroy window error", "Null menu", "Print aborted", "Bad print record", "Print driver error", "Windows error during printing", "Memory error during printing", "Print dialog error", "Generic print error", "Invalid device refnum", "Device not found", "Device parameter error", "Device unit error", "Cannot open device", "Device call aborted", "Generic error", "Cancelled by user", "Object ID too low", "Object ID too high", "Object not in heap", "Unknown heap", "Unknown object (invalid DefProc)", "Unknown object (DefProc not in table)", "Message out of range", "Invalid (null) method", "Unknown message", "Manager call not supported", "Bad address", "Network operation in progress", "Network operation timed out", "Connection is busy", "Network attribute not supported", "Network error", "Address in use", "System out of memory", "Connection aborted", "Connection refused", "Not connected", "Already connected", "Connection closed", "Initialization error (interapplication manager)", "Bad occurrence", "Wait on unbound occurrence handler", "Occurrence queue overflow", "Datalog type conflict", "Unused", "Unrecognized type (interapplication manager)", "Memory corrupt", "Failed to make temporary DLL", "Old CIN version", "Drag socket not found", "Failed to load drop-object", "Failed to register OLE object", "Failed to release OLE object", "Format specifier type mismatch", "Unknown format specifier", "Too few format specifiers", "Too many format specifiers", "Scan failed", "Newer CIN version", "Error converting to variant", "Runtime menu error", "Password tampered", "Variant attribute not found", "Incompatible variant data type", "Event data is not available", "Event Store is not present", "Occurrence is not found", "Event Queue is not created", "Event info is not available", "Refnum passed is NULL", "Error retrieving Class GUID", "Error retrieving CoClass GUID", "Error retrieving TypeLib GUID.", "Bad built application magic bytes.", "Specific driver is different from the specific driver associated with the Logical Name.", "There is no session opened to the class driver.", "Max Error", "MAX - Error with config objects", "MAX - Error loading configuration", "MAX - Group not supported"]
        # "Current State"
        # "Do not delete, rename, or modify this frame.\n(this is used to capture unhandled states and typos)"
        # "Handle mistyped state name (developer tool)"
        n84 = Format Into String(format string="Software Exception: Unhandled State \"%s\"." ("message"), error in=w223, w218) -> (resulting string=w226:string, error out=w225:errorcluster)  [unwired: 1 in]
        n85 = call <vilib>:"Error Cluster From Error Code.vi"("show call chain? (False)"=TRUE, "error in (no error)"=w225, "error message (\"\")"=w226, "error code (0)"=w227) -> ("error out"=w224:errorcluster)  [unwired: 5 in]
        n86 = call <vilib>:"Add State(s) to Queue__JKI_lib_State_Machine.vi"("State(s) in (\"\")"=w222) -> ("States Out"=w221:string)  [unwired: 14 in]
      }
      frame "Initialize Core Data" {
        # "Do not delete, rename, or modify this frame.\n(this is used to determine panel behavior on exit)"
        # "originally closed?"
        # "exe?"
        # "If panel starts closed or is an EXE, then close it when we exit"
        n87 = property class="VI"() -> ("FP.State"=w231:T2)  [unwired: 2 in, 2 out]
        n88 = property class="App"() -> ("App.Kind"=w237:T3)  [unwired: 2 in, 2 out]
        n89 = control-ref of="Current VI Reference"() -> (w232:refnum<vi>)
        n90 = Equal?(x=w231, y=T2."Closed" ("Front Panel Window:State")) -> (x = y?=w229:bool)
        n91 = Equal?(x=w237, y=T3."Run Time System" ("Application:Kind")) -> (x = y?=w235:bool)
        n92 = Or(x=w229, y=w235) -> (x .or. y?=w233:bool)
        n93 = Bundle By Name(cluster=w234, "Core.Current VI Reference"=w232, "Core.Close Panel on Exit?"=w233) -> (w239:T4)
        n94 = call <vilib>:"Add State(s) to Queue__JKI_lib_State_Machine.vi"("State(s) in (\"\")"=w241) -> ("States Out"=w240:string)  [unwired: 14 in]
      }
      frame "Error Handler" {
        # "Unhandled Error -- Display it"
        # "Handle any errors here.\nYou can also output any states to clean-up after errors occur"
        # "Clear error"
        n95 = call <vilib>:"General Error Handler.vi"("error in (no error)"=w243) -> ()  [unwired: 10 in, 5 out]
        n96 = call <vilib>:"Add State(s) to Queue__JKI_lib_State_Machine.vi"("State(s) in Front (\"\")"="/* Post Error States", "State(s) in (\"\")"=w247) -> ("States Out"=w246:string)  [unwired: 13 in]
      }
      frame "Exit" {
        # "Do not put any code in this frame.\n(No errors that occur here will be handled.)"
        n97 = Unbundle By Name(w251) -> ("Rotation Instance"=w249:refnum<class "Modbus Master.lvclass">)
        n98 = call-dynamic "Shutdown.vi"("error in"=w248, "Modbus master in"=w249) -> ("error out"=w250:errorcluster)  [unwired: 9 in]
        n99 = call <vilib>:"Add State(s) to Queue__JKI_lib_State_Machine.vi"("State(s) in (\"\")"=w254) -> ("States Out"=w253:string)  [unwired: 14 in]
      }
      frame "---------- Data ----------" {
        # "Do not put any code in this frame.\n(It is a separator no-op. You can make a copy of this frame to create a new Data frame)"
        n100 = call <vilib>:"Add State(s) to Queue__JKI_lib_State_Machine.vi"("State(s) in (\"\")"=w258) -> ("States Out"=w257:string)  [unwired: 14 in]
      }
      frame "Data: Initialize" {
        w259 = FALSE  # Grease
        w260 = FALSE  # D Shape
        w261 = FALSE  # Tension
        w262 = refnum<class "Modbus Master.lvclass"> refnum  # Rotation Instance
        w264 = T5 {"Current VI Reference"=refnum, "Close Panel on Exit?"=FALSE}  # Core
        # "Initialize the shift-register data, here.\n(data names are defined by what you wire into the bundle function)"
        n101 = Bundle("Core"=w264, "COM Port"="COM Port", "Rotation Instance"=w262, "Tension"=w261, "D Shape"=w260, "Grease"=w259) -> (w266:T4)  [unwired: 1 in]
        n102 = call <vilib>:"Add State(s) to Queue__JKI_lib_State_Machine.vi"("State(s) in (\"\")"=w268) -> ("States Out"=w267:string)  [unwired: 14 in]
      }
      frame "Data: Cleanup" {
        # "Cleanup any data and references, here.\n(this is called automatically, by the Macro: Exit)"
        n103 = Unbundle By Name(w269) -> ("Core.Current VI Reference"=w272:refnum<vi>)
        n104 = Close Reference(reference=w272, error in (no error)=w271) -> (error out=w270:errorcluster)
        n105 = call <vilib>:"Add State(s) to Queue__JKI_lib_State_Machine.vi"("State(s) in (\"\")"=w274) -> ("States Out"=w273:string)  [unwired: 14 in]
      }
      frame "---------- UI ----------" {
        # "Do not put any code in this frame.\n(It is a separator no-op. You can make a copy of this frame to create a new UI frame)"
        n106 = call <vilib>:"Add State(s) to Queue__JKI_lib_State_Machine.vi"("State(s) in (\"\")"=w278) -> ("States Out"=w277:string)  [unwired: 14 in]
      }
      frame "UI: Initialize" {
        w279 = FALSE ("Tension")
        w290 = u16 0 items=["None", "XON/XOFF", "RTS/CTS", "XON/XOFF & RTS/CTS", "DTR/DSR", "XON/XOFF & DTR/DSR"]  # flow control (none)
        w288 = u16 2 items=["None", "Odd", "Even", "Mark", "Space"]  # parity (even)
        w289 = enum16{"RTU", "ASCII"}."RTU"  # serial type
        w281 = u8 1  # unit ID
        # "Initialize the User Interface, here.\n(this is called automatically, by the Macro: Init)"
        n107 = Unbundle By Name(w284) -> ("COM Port"=w285:refnum<visa-resource-name>)
        n108 = call-poly <vilib>:"Create Modbus Instance.vi"("flow control (none)"=w290, "serial type"=w289, "parity (even)"=w288, "unit ID"=w281, "error in"=w286, "baud rate"=u32 9600, "VISA resource name"=w285) -> ("error out"=w280:errorcluster, "serial master instance"=w282:refnum<class "Modbus Master.lvclass">)  [unwired: 3 in]
        n109 = call <vilib>:"Add State(s) to Queue__JKI_lib_State_Machine.vi"("State(s) in (\"\")"=w292) -> ("States Out"=w291:string)  [unwired: 14 in]
        n110 = local write "Tension"(w279) -> ()
        n111 = local write "D-Shape"(w279) -> ()
        n112 = local write "Grease"(w279) -> ()
        n113 = Bundle By Name(cluster=w284, "Rotation Instance"=w282) -> (w283:T4)
      }
      frame "UI: Cursor Set" {
        # "Argument"
        # "Set and Unset Cursor Busy.\n(Usage: \"UI: Cursor Set >> Busy|Idle\")"
        n114 = case shown="\"Idle\", Default" w293 {
          tunnel: w295 -> [w300 w302]
          tunnel: [w299 w301] -> w294
          frame "Idle", Default {
            n115 = call <vilib>:"Unset Busy.vi"("error in (no error)"=w300) -> ("error out"=w299:errorcluster)  [unwired: 10 in]
          }
          frame "Busy" {
            n116 = call <vilib>:"Set Busy.vi"("error in (no error)"=w302) -> ("error out"=w301:errorcluster)  [unwired: 9 in, 1 out]
          }
        }
        n117 = call <vilib>:"Add State(s) to Queue__JKI_lib_State_Machine.vi"("State(s) in (\"\")"=w298) -> ("States Out"=w297:string)  [unwired: 14 in]
      }
      frame "UI: Front Panel State" {
        # "Argument"
        # "Set Front Panel Open or Closed\n(Usage: \"UI: Front Panel State >> Open|Close\")"
        n118 = Unbundle By Name(w305) -> ("Core.Current VI Reference"=w304:refnum<vi>)
        n119 = case shown="\"Minimize\", \"Minimized\"" w303 {
          tunnel: w307 -> [w315 w330 w341 w354 w367]
          tunnel: [w317 w331 w343 w356 w369] -> w306
          tunnel: w304 -> [w316 w328 w342 w355 w368]
          frame "Open", "Standard", Default {
            w310 = T2."Standard" ("State")
            n120 = property class="VI"(reference=w316, error in=w315) -> (reference out=w313:refnum<vi>, error out=w314:errorcluster, "FP.State"=w312:T2)
            n121 = Not Equal?(x=w312, y=w310) -> (x != y?=w311:bool)
            n122 = case shown="True" w311 {
              tunnel: [w321 w323] -> w317
              tunnel: w314 -> [w320 w323]
              tunnel: w313 -> [w319 _]
              tunnel: w310 -> [w318 _]
              frame True {
                n123 = invoke class="VI" method="FP.Open"(reference=w319, error in=w320, "Activate"=TRUE, "State"=w318) -> (error out=w321:errorcluster)  [unwired: 1 in, 4 out]
              }
              frame False {
              }
            }
          }
          frame "Close", "Closed" {
            n124 = property class="VI"(reference=w328, error in=w330) -> (reference out=w327:refnum<vi>, error out=w329:errorcluster, "FP.State"=w325:T2)
            n125 = Not Equal?(x=w325, y=T2."Closed" ("Front Panel Window:State")) -> (x != y?=w324:bool)
            n126 = case shown="True" w324 {
              tunnel: [w332 w335] -> w331
              tunnel: w329 -> [w332 w334]
              tunnel: w327 -> [_ w333]
              frame False {
              }
              frame True {
                n127 = invoke class="VI" method="FP.Close"(reference=w333, error in=w334) -> (error out=w335:errorcluster)  [unwired: 1 in, 2 out]
              }
            }
          }
          frame "Hidden", "Hide" {
            w336 = T2."Hidden" ("State")
            n128 = property class="VI"(reference=w342, error in=w341) -> (reference out=w339:refnum<vi>, error out=w340:errorcluster, "FP.State"=w338:T2)
            n129 = Not Equal?(x=w338, y=w336) -> (x != y?=w337:bool)
            n130 = case shown="True" w337 {
              tunnel: [w347 w348] -> w343
              tunnel: w340 -> [w346 w348]
              tunnel: w339 -> [w345 _]
              tunnel: w336 -> [w344 _]
              frame True {
                n131 = invoke class="VI" method="FP.Open"(reference=w345, error in=w346, "State"=w344) -> (error out=w347:errorcluster)  [unwired: 2 in, 4 out]
              }
              frame False {
              }
            }
          }
          frame "Minimize", "Minimized" {
            w349 = T2."Minimized" ("State")
            n132 = property class="VI"(reference=w355, error in=w354) -> (reference out=w352:refnum<vi>, error out=w353:errorcluster, "FP.State"=w351:T2)
            n133 = Not Equal?(x=w351, y=w349) -> (x != y?=w350:bool)
            n134 = case shown="True" w350 {
              tunnel: [w360 w361] -> w356
              tunnel: w353 -> [w359 w361]
              tunnel: w352 -> [w358 _]
              tunnel: w349 -> [w357 _]
              frame True {
                n135 = invoke class="VI" method="FP.Open"(reference=w358, error in=w359, "State"=w357) -> (error out=w360:errorcluster)  [unwired: 2 in, 4 out]
              }
              frame False {
              }
            }
          }
          frame "Maximize", "Maximized" {
            w362 = T2."Maximized" ("State")
            n136 = property class="VI"(reference=w368, error in=w367) -> (reference out=w365:refnum<vi>, error out=w366:errorcluster, "FP.State"=w364:T2)
            n137 = Not Equal?(x=w364, y=w362) -> (x != y?=w363:bool)
            n138 = case shown="True" w363 {
              tunnel: [w373 w374] -> w369
              tunnel: w366 -> [w372 w374]
              tunnel: w365 -> [w371 _]
              tunnel: w362 -> [w370 _]
              frame True {
                n139 = invoke class="VI" method="FP.Open"(reference=w371, error in=w372, "State"=w370) -> (error out=w373:errorcluster)  [unwired: 2 in, 4 out]
              }
              frame False {
              }
            }
          }
        }
        n140 = call <vilib>:"Add State(s) to Queue__JKI_lib_State_Machine.vi"("State(s) in (\"\")"=w309) -> ("States Out"=w308:string)  [unwired: 14 in]
      }
      frame "---------- Macro ----------" {
        # "Do not put any code in this frame.\n(It is a separator no-op. You can make a copy of this frame to create a new Macro frame)"
        n141 = call <vilib>:"Add State(s) to Queue__JKI_lib_State_Machine.vi"("State(s) in (\"\")"=w378) -> ("States Out"=w377:string)  [unwired: 14 in]
      }
      frame "Macro: Initialize" {
        w379 = "Data: Initialize\nInitialize Core Data\nUI: Initialize\nUI: Front Panel State >> Open"  # Data: Initialize Initialize Core Data UI: Initialize UI: Front Panel State >> Open
        # "Initialization Macro\n(This is called once, when the VI starts)"
        n142 = call <vilib>:"Add State(s) to Queue__JKI_lib_State_Machine.vi"("State(s) in Front (\"\")"=w379, "State(s) in (\"\")"=w383) -> ("States Out"=w382:string)  [unwired: 13 in]
      }
      frame "Macro: Exit" {
        # "Exit Macro\n(This is called once, when the VI exits)"
        n143 = Unbundle By Name(w390) -> ("Core.Close Panel on Exit?"=w389:bool)
        n144 = Select(t="UI: Front Panel State >> Close", s=w389, f="") -> (s? t:f=w386:string)
        n145 = call <vilib>:"Add State(s) to Queue__JKI_lib_State_Machine.vi"("State(s) in (\"\")"=w386, "State(s) at Back (\"\")"="Data: Cleanup\nExit") -> ("States Out"=w384:string)  [unwired: 13 in]
        n146 = call <vilib>:"Add State(s) to Queue__JKI_lib_State_Machine.vi"("State(s) in Front (\"\")"=w384, "State(s) in (\"\")"=w393) -> ("States Out"=w392:string)  [unwired: 13 in]
      }
      frame "---------- New Category ----------" {
        # "Template Separator\n(You can make a copy of, or modify, this frame)"
        n147 = call <vilib>:"Add State(s) to Queue__JKI_lib_State_Machine.vi"("State(s) in (\"\")"=w397) -> ("States Out"=w396:string)  [unwired: 14 in]
      }
      frame "Sequence 0" {
        n148 = Unbundle By Name(w399) -> ("Rotation Instance"=w407:refnum<class "Modbus Master.lvclass">)
        n149 = call "E700-Sequence.vi"("Direction Switch"="Seq 0 Direction Switch", "Rotation Instance"=w407, "error in (no error)"=w408, "Time (mS) - Seq 1"="Time (mS) - Seq 0", "Vertical Frequencey Setting (Hz) - Seq 1"="Vertical Frequencey Setting (Hz) - Seq 0", "Rotational Frequencey Setting (Hz) - Seq 1"="Rotational Frequencey Setting (Hz) - Seq 0") -> ("error out"=w401:errorcluster)  [unwired: 9 in]
        n150 = local write "Status"("Sequence 0 - Tension Offset and Start D at END" ("Status")) -> ()
        n151 = flat-sequence {
          tunnel: w401 -> [w414]
          tunnel: [w414] -> w400
          tunnel: w399 -> [w413]
          tunnel: [w412] -> w398
          frame #0 {
            w411 = TRUE ("D Shape")
            n152 = Bundle By Name(cluster=w413, "D Shape"=w411) -> (w412:T4)
            "D-Shape" <- w411
          }
        }
        n153 = call <vilib>:"Add State(s) to Queue__JKI_lib_State_Machine.vi"("State(s) in (\"\")"=w410) -> ("States Out"=w409:string)  [unwired: 14 in]
      }
      frame "Sequence 1" {
        n154 = Unbundle By Name(w415) -> ("Rotation Instance"=w424:refnum<class "Modbus Master.lvclass">)
        n155 = local write "Status"("Sequence 1 - Start Grease at END" ("Status")) -> ()
        n156 = call "E700-Sequence.vi"("Direction Switch"="Seq 1 Direction Switch", "Rotation Instance"=w424, "error in (no error)"=w425, "Time (mS) - Seq 1"="Time (mS) - Seq 1", "Vertical Frequencey Setting (Hz) - Seq 1"="Vertical Frequencey Setting (Hz) - Seq 1", "Rotational Frequencey Setting (Hz) - Seq 1"="Rotational Frequencey Setting (Hz) - Seq 1") -> ("error out"=w418:errorcluster)  [unwired: 9 in]
        n157 = flat-sequence {
          tunnel: w418 -> [w431]
          tunnel: [w431] -> w417
          tunnel: w415 -> [w430]
          tunnel: [w429] -> w416
          frame #0 {
            w428 = TRUE ("Grease")
            n158 = Bundle By Name(cluster=w430, "Grease"=w428) -> (w429:T4)
            "Grease" <- w428
          }
        }
        n159 = call <vilib>:"Add State(s) to Queue__JKI_lib_State_Machine.vi"("State(s) in (\"\")"=w427) -> ("States Out"=w426:string)  [unwired: 14 in]
      }
      frame "Sequence 2" {
        n160 = Unbundle By Name(w432) -> ("Rotation Instance"=w440:refnum<class "Modbus Master.lvclass">)
        n161 = call "E700-Sequence.vi"("Direction Switch"="Seq 2 Direction Switch", "Rotation Instance"=w440, "error in (no error)"=w441, "Time (mS) - Seq 1"="Time (mS) - Seq 2", "Vertical Frequencey Setting (Hz) - Seq 1"="Vertical Frequencey Setting (Hz) - Seq 2", "Rotational Frequencey Setting (Hz) - Seq 1"="Rotational Frequencey Setting (Hz) - Seq 2") -> ("error out"=w435:errorcluster)  [unwired: 9 in]
        n162 = flat-sequence {
          tunnel: w435 -> [w448]
          tunnel: [w448] -> w434
          tunnel: w432 -> [w447]
          tunnel: [w446] -> w433
          frame #0 {
            w445 = TRUE ("Tension")
            n163 = Bundle By Name(cluster=w447, "Tension"=w445) -> (w446:T4)
            "Tension" <- w445
          }
        }
        n164 = call <vilib>:"Add State(s) to Queue__JKI_lib_State_Machine.vi"("State(s) in (\"\")"=w444) -> ("States Out"=w443:string)  [unwired: 14 in]
        "Status" <- "Sequence 2 - Install Clamp at END and Turn Tension ON at END" ("Status")
      }
      frame "Sequence 3" {
        n165 = Unbundle By Name(w457) -> ("Rotation Instance"=w454:refnum<class "Modbus Master.lvclass">)
        n166 = call "E700-Sequence.vi"("Direction Switch"="Seq 3 Direction Switch", "Rotation Instance"=w454, "error in (no error)"=w456, "Time (mS) - Seq 1"="Time (mS) - Seq 3", "Vertical Frequencey Setting (Hz) - Seq 1"="Vertical Frequencey Setting (Hz) - Seq 3", "Rotational Frequencey Setting (Hz) - Seq 1"="Rotational Frequencey Setting (Hz) - Seq 3") -> ("error out"=w455:errorcluster)  [unwired: 9 in]
        n167 = local write "Status"("Sequence 3 - Three Revolutions" ("Status")) -> ()
        n168 = call <vilib>:"Add State(s) to Queue__JKI_lib_State_Machine.vi"("State(s) in (\"\")"=w459) -> ("States Out"=w458:string)  [unwired: 14 in]
      }
      frame "Sequence 4" {
        n169 = flat-sequence {
          tunnel: w463 -> [w476]
          tunnel: [w476] -> w462
          tunnel: w464 -> [w475]
          tunnel: [w474] -> w460
          frame #0 {
            w473 = FALSE ("Grease")
            n170 = Bundle By Name(cluster=w475, "Grease"=w473) -> (w474:T4)
            n171 = local write "Grease"(w473) -> ()
          }
        }
        n172 = Unbundle By Name(w460) -> ("Rotation Instance"=w467:refnum<class "Modbus Master.lvclass">)
        n173 = local write "Status"("Sequence 4 - Vertical Drop" ("Status")) -> ()
        n174 = call "E700-Sequence.vi"("Direction Switch"="Seq 4 Direction Switch", "Rotation Instance"=w467, "error in (no error)"=w462, "Time (mS) - Seq 1"="Time (mS) - Seq 4", "Vertical Frequencey Setting (Hz) - Seq 1"="Vertical Frequencey Setting (Hz) - Seq 4", "Rotational Frequencey Setting (Hz) - Seq 1"="Rotational Frequencey Setting (Hz) - Seq 4") -> ("error out"=w461:errorcluster)  [unwired: 9 in]
        n175 = call <vilib>:"Add State(s) to Queue__JKI_lib_State_Machine.vi"("State(s) in (\"\")"=w472) -> ("States Out"=w471:string)  [unwired: 14 in]
      }
      frame "Sequence 5" {
        n176 = flat-sequence {
          tunnel: w479 -> [w493]
          tunnel: [w493] -> w480
          tunnel: w481 -> [w492]
          tunnel: [w491] -> w478
          frame #0 {
            w490 = TRUE ("Grease")
            n177 = Bundle By Name(cluster=w492, "Grease"=w490) -> (w491:T4)
            n178 = local write "Grease"(w490) -> ()
          }
        }
        n179 = Unbundle By Name(w478) -> ("Rotation Instance"=w487:refnum<class "Modbus Master.lvclass">)
        n180 = call "E700-Sequence.vi"("Direction Switch"="Seq 5 Direction Switch", "Rotation Instance"=w487, "error in (no error)"=w480, "Time (mS) - Seq 1"="Time (mS) - Seq 5", "Vertical Frequencey Setting (Hz) - Seq 1"="Vertical Frequencey Setting (Hz) - Seq 5", "Rotational Frequencey Setting (Hz) - Seq 1"="Rotational Frequencey Setting (Hz) - Seq 5") -> ("error out"=w477:errorcluster)  [unwired: 9 in]
        n181 = local write "Status"("Sequence 5 - 3/4 Turn Offset" ("Status")) -> ()
        n182 = call <vilib>:"Add State(s) to Queue__JKI_lib_State_Machine.vi"("State(s) in (\"\")"=w489) -> ("States Out"=w488:string)  [unwired: 14 in]
      }
      frame "Sequence 6" {
        n183 = Unbundle By Name(w502) -> ("Rotation Instance"=w497:refnum<class "Modbus Master.lvclass">)
        n184 = call "E700-Sequence.vi"("Direction Switch"="Seq 6 Direction Switch", "Rotation Instance"=w497, "error in (no error)"=w501, "Time (mS) - Seq 1"="Time (mS) - Seq 6", "Vertical Frequencey Setting (Hz) - Seq 1"="Vertical Frequencey Setting (Hz) - Seq 6", "Rotational Frequencey Setting (Hz) - Seq 1"="Rotational Frequencey Setting (Hz) - Seq 6") -> ("error out"=w496:errorcluster)  [unwired: 9 in]
        n185 = local write "Status"("Sequence 6 - Four Revolutions" ("Status")) -> ()
        n186 = call <vilib>:"Add State(s) to Queue__JKI_lib_State_Machine.vi"("State(s) in (\"\")"=w504) -> ("States Out"=w503:string)  [unwired: 14 in]
      }
      frame "Sequence 7" {
        n187 = flat-sequence {
          tunnel: w507 -> [w521]
          tunnel: [w521] -> w506
          tunnel: w509 -> [w520]
          tunnel: [w519] -> w508
          frame #0 {
            w518 = FALSE ("Grease")
            n188 = Bundle By Name(cluster=w520, "Grease"=w518) -> (w519:T4)
            n189 = local write "Grease"(w518) -> ()
          }
        }
        n190 = Unbundle By Name(w508) -> ("Rotation Instance"=w515:refnum<class "Modbus Master.lvclass">)
        n191 = local write "Status"("Sequence 7 - Vertical Drop" ("Status")) -> ()
        n192 = call "E700-Sequence.vi"("Direction Switch"="Seq 7 Direction Switch", "Rotation Instance"=w515, "error in (no error)"=w506, "Time (mS) - Seq 1"="Time (mS) - Seq 7", "Vertical Frequencey Setting (Hz) - Seq 1"="Vertical Frequencey Setting (Hz) - Seq 7", "Rotational Frequencey Setting (Hz) - Seq 1"="Rotational Frequencey Setting (Hz) - Seq 7") -> ("error out"=w505:errorcluster)  [unwired: 9 in]
        n193 = call <vilib>:"Add State(s) to Queue__JKI_lib_State_Machine.vi"("State(s) in (\"\")"=w517) -> ("States Out"=w516:string)  [unwired: 14 in]
      }
      frame "Sequence 8" {
        n194 = flat-sequence {
          tunnel: w523 -> [w538]
          tunnel: [w538] -> w524
          tunnel: w526 -> [w537]
          tunnel: [w536] -> w525
          frame #0 {
            w535 = TRUE ("Grease")
            n195 = Bundle By Name(cluster=w537, "Grease"=w535) -> (w536:T4)
            n196 = local write "Grease"(w535) -> ()
          }
        }
        n197 = Unbundle By Name(w525) -> ("Rotation Instance"=w532:refnum<class "Modbus Master.lvclass">)
        n198 = local write "Status"("Sequence 8 - 3/4 Turn Offset" ("Status")) -> ()
        n199 = call "E700-Sequence.vi"("Direction Switch"="Seq 8 Direction Switch", "Rotation Instance"=w532, "error in (no error)"=w524, "Time (mS) - Seq 1"="Time (mS) - Seq 8", "Vertical Frequencey Setting (Hz) - Seq 1"="Vertical Frequencey Setting (Hz) - Seq 8", "Rotational Frequencey Setting (Hz) - Seq 1"="Rotational Frequencey Setting (Hz) - Seq 8") -> ("error out"=w522:errorcluster)  [unwired: 9 in]
        n200 = call <vilib>:"Add State(s) to Queue__JKI_lib_State_Machine.vi"("State(s) in (\"\")"=w534) -> ("States Out"=w533:string)  [unwired: 14 in]
      }
      frame "Sequence 9" {
        n201 = Unbundle By Name(w547) -> ("Rotation Instance"=w545:refnum<class "Modbus Master.lvclass">)
        n202 = call "E700-Sequence.vi"("Direction Switch"="Seq 9 Direction Switch", "Rotation Instance"=w545, "error in (no error)"=w546, "Time (mS) - Seq 1"="Time (mS) - Seq 9", "Vertical Frequencey Setting (Hz) - Seq 1"="Vertical Frequencey Setting (Hz) - Seq 9", "Rotational Frequencey Setting (Hz) - Seq 1"="Rotational Frequencey Setting (Hz) - Seq 9") -> ("error out"=w544:errorcluster)  [unwired: 9 in]
        n203 = local write "Status"("Sequence 9 - Three Revolutions" ("Status")) -> ()
        n204 = call <vilib>:"Add State(s) to Queue__JKI_lib_State_Machine.vi"("State(s) in (\"\")"=w549) -> ("States Out"=w548:string)  [unwired: 14 in]
      }
      frame "Sequence 10" {
        n205 = Unbundle By Name(w558) -> ("Rotation Instance"=w556:refnum<class "Modbus Master.lvclass">)
        n206 = call "E700-Sequence.vi"("Direction Switch"="Seq 10 Direction Switch", "Rotation Instance"=w556, "error in (no error)"=w557, "Time (mS) - Seq 1"="Time (mS) - Seq 10", "Vertical Frequencey Setting (Hz) - Seq 1"="Vertical Frequencey Setting (Hz) - Seq 10", "Rotational Frequencey Setting (Hz) - Seq 1"="Rotational Frequencey Setting (Hz) - Seq 10") -> ("error out"=w555:errorcluster)  [unwired: 9 in]
        n207 = local write "Status"("Sequence 10 - Nine Revolutions" ("Status")) -> ()
        n208 = call <vilib>:"Add State(s) to Queue__JKI_lib_State_Machine.vi"("State(s) in (\"\")"=w560) -> ("States Out"=w559:string)  [unwired: 14 in]
      }
      frame "Sequence 11" {
        n209 = flat-sequence {
          tunnel: w563 -> [w577]
          tunnel: [w577] -> w562
          tunnel: w565 -> [w576]
          tunnel: [w575] -> w564
          frame #0 {
            w574 = FALSE ("Grease")
            n210 = Bundle By Name(cluster=w576, "Grease"=w574) -> (w575:T4)
            n211 = local write "Grease"(w574) -> ()
          }
        }
        n212 = Unbundle By Name(w564) -> ("Rotation Instance"=w571:refnum<class "Modbus Master.lvclass">)
        n213 = call "E700-Sequence.vi"("Direction Switch"="Seq 11 Direction Switch", "Rotation Instance"=w571, "error in (no error)"=w562, "Time (mS) - Seq 1"="Time (mS) - Seq 11", "Vertical Frequencey Setting (Hz) - Seq 1"="Vertical Frequencey Setting (Hz) - Seq 11", "Rotational Frequencey Setting (Hz) - Seq 1"="Rotational Frequencey Setting (Hz) - Seq 11") -> ("error out"=w561:errorcluster)  [unwired: 9 in]
        n214 = local write "Status"("Sequence 11 - Vertical Drop" ("Status")) -> ()
        n215 = call <vilib>:"Add State(s) to Queue__JKI_lib_State_Machine.vi"("State(s) in (\"\")"=w573) -> ("States Out"=w572:string)  [unwired: 14 in]
      }
      frame "Sequence 12" {
        n216 = flat-sequence {
          tunnel: w579 -> [w596]
          tunnel: [w596] -> w578
          tunnel: w581 -> [w595]
          tunnel: [w594] -> w580
          frame #0 {
            w593 = TRUE ("Grease")
            n217 = Bundle By Name(cluster=w595, "Grease"=w593) -> (w594:T4)
            n218 = local write "Grease"(w593) -> ()
          }
        }
        n219 = Unbundle By Name(w580) -> ("Rotation Instance"=w590:refnum<class "Modbus Master.lvclass">)
        n220 = call "E700-Sequence.vi"("Direction Switch"="Seq 12 Direction Switch", "Rotation Instance"=w590, "error in (no error)"=w578, "Time (mS) - Seq 1"="Time (mS) - Seq 12", "Vertical Frequencey Setting (Hz) - Seq 1"="Vertical Frequencey Setting (Hz) - Seq 12", "Rotational Frequencey Setting (Hz) - Seq 1"="Rotational Frequencey Setting (Hz) - Seq 12") -> ("error out"=w584:errorcluster)  [unwired: 9 in]
        n221 = flat-sequence {
          tunnel: w584 -> [w600]
          tunnel: [w600] -> w583
          tunnel: w581 -> [w599]
          tunnel: [w598] -> w582
          frame #0 {
            w597 = FALSE ("D Shape")
            n222 = local write "D-Shape"(w597) -> ()
            n223 = Bundle By Name(cluster=w599, "D Shape"=w597) -> (w598:T4)
          }
        }
        n224 = call <vilib>:"Add State(s) to Queue__JKI_lib_State_Machine.vi"("State(s) in (\"\")"=w592) -> ("States Out"=w591:string)  [unwired: 14 in]
        n225 = local write "Status"("Sequence 12 - One Revolution + 45 Degrees - Turn D off at END " ("Status")) -> ()
      }
      frame "Sequence 13" {
        n226 = Unbundle By Name(w603) -> ("Rotation Instance"=w610:refnum<class "Modbus Master.lvclass">)
        n227 = call "E700-Sequence.vi"("Direction Switch"="Seq 13 Direction Switch", "Rotation Instance"=w610, "error in (no error)"=w611, "Time (mS) - Seq 1"="Time (mS) - Seq 13", "Vertical Frequencey Setting (Hz) - Seq 1"="Vertical Frequencey Setting (Hz) - Seq 13", "Rotational Frequencey Setting (Hz) - Seq 1"="Rotational Frequencey Setting (Hz) - Seq 13") -> ("error out"=w602:errorcluster)  [unwired: 9 in]
        n228 = local write "Status"("Sequence 13 - 100 Degree Revolution, Turn Grease off at END" ("Status")) -> ()
        n229 = flat-sequence {
          tunnel: w603 -> [w617]
          tunnel: [w616] -> w604
          tunnel: w602 -> [w615]
          tunnel: [w615] -> w601
          frame #0 {
            w614 = FALSE ("Grease")
            n230 = Bundle By Name(cluster=w617, "Grease"=w614) -> (w616:T4)
            n231 = local write "Grease"(w614) -> ()
          }
        }
        n232 = call <vilib>:"Add State(s) to Queue__JKI_lib_State_Machine.vi"("State(s) in (\"\")"=w613) -> ("States Out"=w612:string)  [unwired: 14 in]
      }
      frame "Sequence 14" {
        n233 = Unbundle By Name(w619) -> ("Rotation Instance"=w627:refnum<class "Modbus Master.lvclass">)
        n234 = call "E700-Sequence.vi"("Direction Switch"="Seq 14 Direction Switch", "Rotation Instance"=w627, "error in (no error)"=w628, "Time (mS) - Seq 1"="Time (mS) - Seq 14", "Vertical Frequencey Setting (Hz) - Seq 1"="Vertical Frequencey Setting (Hz) - Seq 14", "Rotational Frequencey Setting (Hz) - Seq 1"="Rotational Frequencey Setting (Hz) - Seq 14") -> ("error out"=w621:errorcluster)  [unwired: 9 in]
        n235 = flat-sequence {
          tunnel: w621 -> [w632]
          tunnel: w619 -> [w634]
          tunnel: [w633] -> w620
          tunnel: [w632] -> w618
          frame #0 {
            w631 = FALSE ("Tension")
            n236 = Bundle By Name(cluster=w634, "Tension"=w631) -> (w633:T4)
            n237 = local write "Tension"(w631) -> ()
          }
        }
        n238 = local write "Status"("Sequence 14 - Finish Revolution and Install Clamp and Turn Tension OFF at END" ("Status")) -> ()
        n239 = call <vilib>:"Add State(s) to Queue__JKI_lib_State_Machine.vi"("State(s) in (\"\")"=w630) -> ("States Out"=w629:string)  [unwired: 14 in]
      }
      frame "Sequence 15" {
        n240 = Unbundle By Name(w643) -> ("Rotation Instance"=w641:refnum<class "Modbus Master.lvclass">)
        n241 = local write "Status"("Sequence 15 - Create Tail" ("Status")) -> ()
        n242 = call "E700-Sequence.vi"("Direction Switch"="Seq 15 Direction Switch", "Rotation Instance"=w641, "error in (no error)"=w642, "Time (mS) - Seq 1"="Time (mS) - Seq 15", "Vertical Frequencey Setting (Hz) - Seq 1"="Vertical Frequencey Setting (Hz) - Seq 15", "Rotational Frequencey Setting (Hz) - Seq 1"="Rotational Frequencey Setting (Hz) - Seq 15") -> ("error out"=w640:errorcluster)  [unwired: 9 in]
        n243 = call <vilib>:"Add State(s) to Queue__JKI_lib_State_Machine.vi"("State(s) in (\"\")"=w645) -> ("States Out"=w644:string)  [unwired: 14 in]
      }
      frame "Read_Data" {
        # "Your code here.\n(You can make a copy of, or modify, this frame)"
        n244 = disable-structure shown="Enabled" {
          disable-tunnel: w648 -> [w664 _]
          disable-tunnel: w647 -> [w654 w672]
          disable-tunnel: [w651 w672] -> w646
          frame Disabled {
            n245 = Unbundle By Name(w664) -> ("Rotation Instance"=w656:refnum<class "Modbus Master.lvclass">, "Vertical Instance"=w655)
            n246 = call-dynamic "Read Holding Registers.vi"("error in"=w654, "number of inputs"=u16 1, "starting address"=u16 200, "Modbus master in"=w656) -> ("error out"=w653:errorcluster, "register values"=w668:u16[])  [unwired: 5 in, 1 out]
            n247 = call-dynamic "Read Holding Registers.vi"("error in"=w654, "number of inputs"=u16 1, "starting address"=u16 200, "Modbus master in"=w655) -> ("error out"=w652:errorcluster, "register values"=w660:u16[])  [unwired: 5 in, 1 out]
            n248 = Array To Cluster(array=w668) -> (cluster=w669:T6)
            n249 = Array To Cluster(array=w660) -> (cluster=w659:T6)
            n250 = Unbundle By Name(w669) -> ("register values[0]"=w670:u16)
            n251 = Unbundle By Name(w659) -> ("register values[0]"=w658:u16)
            n252 = Divide(x=w670, y=u16 100) -> (x/y=→"Rotational Frequency Output":dbl)
            n253 = Divide(x=w658, y=u16 100) -> (x/y=→"Vertical Frequency Output":dbl)
            n254 = Merge Errors(w653, w652) -> (w651:errorcluster)
          }
          frame Enabled {
          }
        }
        n255 = call <vilib>:"Add State(s) to Queue__JKI_lib_State_Machine.vi"("State(s) in (\"\")"=w650) -> ("States Out"=w649:string)  [unwired: 14 in]
      }
      frame "Set Rotational Frequency" {
        n256 = Unbundle By Name(w681) -> ("Rotation Instance"=w675:refnum<class "Modbus Master.lvclass">)
        n257 = call "E700-Frequency Setting.vi"("error in (no error)"=w683, "Frequencey Setting (Hz)"="Rotational Frequencey Setting (Hz) - Manual 1") -> ("error out"=w677:errorcluster, "Set Value"=w685:u16)  [unwired: 8 in]
        n258 = call <vilib>:"Set Unit ID.vi"("error in"=w677, "unit ID"=u8 1, "Modbus master in"=w675) -> ("error out"=w676:errorcluster, "Modbus master out"=w674:refnum<class "Modbus Master.lvclass">)  [unwired: 7 in]
        n259 = call-dynamic "Write Single Holding Register.vi"("error in"=w676, "register to write"=w685, "address"=u16 13, "Modbus master in"=w674) -> ("error out"=w682:errorcluster, "Modbus master out"=w679:refnum<class "Modbus Master.lvclass">)  [unwired: 6 in]
        n260 = Bundle By Name(cluster=w681, "Rotation Instance"=w679) -> (w680:T4)
        n261 = call <vilib>:"Add State(s) to Queue__JKI_lib_State_Machine.vi"("State(s) in (\"\")"=w687) -> ("States Out"=w686:string)  [unwired: 14 in]
      }
      frame "Set Rotational Frequency Comb" {
        n262 = Unbundle By Name(w696) -> ("Rotation Instance"=w691:refnum<class "Modbus Master.lvclass">)
        n263 = call "E700-Frequency Setting.vi"("error in (no error)"=w698, "Frequencey Setting (Hz)"="Rotational Frequencey Setting (Hz) - Manual 2") -> ("error out"=w693:errorcluster, "Set Value"=w700:u16)  [unwired: 8 in]
        n264 = call <vilib>:"Set Unit ID.vi"("error in"=w693, "unit ID"=u8 1, "Modbus master in"=w691) -> ("error out"=w692:errorcluster, "Modbus master out"=w690:refnum<class "Modbus Master.lvclass">)  [unwired: 7 in]
        n265 = call-dynamic "Write Single Holding Register.vi"("error in"=w692, "register to write"=w700, "address"=u16 13, "Modbus master in"=w690) -> ("error out"=w697:errorcluster, "Modbus master out"=w694:refnum<class "Modbus Master.lvclass">)  [unwired: 6 in]
        n266 = Bundle By Name(cluster=w696, "Rotation Instance"=w694) -> (w695:T4)
        n267 = call <vilib>:"Add State(s) to Queue__JKI_lib_State_Machine.vi"("State(s) in (\"\")"=w702) -> ("States Out"=w701:string)  [unwired: 14 in]
      }
      frame "Stop Rotational Frequency" {
        n268 = Unbundle By Name(w711) -> ("Rotation Instance"=w704:refnum<class "Modbus Master.lvclass">)
        n269 = call "E700-Frequency Setting.vi"("error in (no error)"=w713, "Frequencey Setting (Hz)"=0.0) -> ("error out"=w706:errorcluster, "Set Value"=w715:u16)  [unwired: 8 in]
        n270 = call <vilib>:"Set Unit ID.vi"("error in"=w706, "unit ID"=u8 1, "Modbus master in"=w704) -> ("error out"=w705:errorcluster, "Modbus master out"=w703:refnum<class "Modbus Master.lvclass">)  [unwired: 7 in]
        n271 = call-dynamic "Write Single Holding Register.vi"("error in"=w705, "register to write"=w715, "address"=u16 13, "Modbus master in"=w703) -> ("error out"=w712:errorcluster, "Modbus master out"=w709:refnum<class "Modbus Master.lvclass">)  [unwired: 6 in]
        n272 = Bundle By Name(cluster=w711, "Rotation Instance"=w709) -> (w710:T4)
        n273 = call <vilib>:"Add State(s) to Queue__JKI_lib_State_Machine.vi"("State(s) in (\"\")"=w717) -> ("States Out"=w716:string)  [unwired: 14 in]
      }
      frame "Set Vertical Frequency" {
        n274 = Unbundle By Name(w730) -> ("Rotation Instance"=w723:refnum<class "Modbus Master.lvclass">)
        n275 = call <vilib>:"Set Unit ID.vi"("error in"=w722, "unit ID"=u8 2, "Modbus master in"=w723) -> ("error out"=w721:errorcluster, "Modbus master out"=w720:refnum<class "Modbus Master.lvclass">)  [unwired: 7 in]
        n276 = call "E700-Inverter Control.vi"("error in (no error)"=w721, "Direction Switch"="Vertical Direction Switch", "ON/OFF - Switch"=TRUE, "Modbus Master in"=w720) -> ("error out"=w727:errorcluster, "Modbus Master out"=w728:refnum<class "Modbus Master.lvclass">)  [unwired: 6 in]
        n277 = call "E700-Frequency Setting.vi"("error in (no error)"=w727, "Frequencey Setting (Hz)"="Vertical Frequencey Setting (Hz) - Manual 1") -> ("error out"=w733:errorcluster, "Set Value"=w734:u16)  [unwired: 8 in]
        n278 = call-dynamic "Write Single Holding Register.vi"("error in"=w733, "register to write"=w734, "address"=u16 13, "Modbus master in"=w728) -> ("error out"=w718:errorcluster, "Modbus master out"=w719:refnum<class "Modbus Master.lvclass">)  [unwired: 6 in]
        n279 = call <vilib>:"Add State(s) to Queue__JKI_lib_State_Machine.vi"("State(s) in (\"\")"=w736) -> ("States Out"=w735:string)  [unwired: 14 in]
        n280 = Bundle By Name(cluster=w730, "Rotation Instance"=w719) -> (w731:T4)
      }
      frame "Set Vertical Frequency Comb" {
        n281 = Unbundle By Name(w749) -> ("Rotation Instance"=w744:refnum<class "Modbus Master.lvclass">)
        n282 = call <vilib>:"Set Unit ID.vi"("error in"=w743, "unit ID"=u8 2, "Modbus master in"=w744) -> ("error out"=w742:errorcluster, "Modbus master out"=w741:refnum<class "Modbus Master.lvclass">)  [unwired: 7 in]
        n283 = call "E700-Inverter Control.vi"("error in (no error)"=w742, "Direction Switch"="Vertical Direction Switch 2", "ON/OFF - Switch"=TRUE, "Modbus Master in"=w741) -> ("error out"=w747:errorcluster, "Modbus Master out"=w748:refnum<class "Modbus Master.lvclass">)  [unwired: 6 in]
        n284 = call "E700-Frequency Setting.vi"("error in (no error)"=w747, "Frequencey Setting (Hz)"="Vertical Frequencey Setting (Hz) - Manual 2") -> ("error out"=w752:errorcluster, "Set Value"=w753:u16)  [unwired: 8 in]
        n285 = call-dynamic "Write Single Holding Register.vi"("error in"=w752, "register to write"=w753, "address"=u16 13, "Modbus master in"=w748) -> ("error out"=w739:errorcluster, "Modbus master out"=w740:refnum<class "Modbus Master.lvclass">)  [unwired: 6 in]
        n286 = call <vilib>:"Add State(s) to Queue__JKI_lib_State_Machine.vi"("State(s) in (\"\")"=w755) -> ("States Out"=w754:string)  [unwired: 14 in]
        n287 = Bundle By Name(cluster=w749, "Rotation Instance"=w740) -> (w750:T4)
      }
      frame "Stop Vertical Frequency" {
        n288 = Unbundle By Name(w764) -> ("Rotation Instance"=w756:refnum<class "Modbus Master.lvclass">)
        n289 = call <vilib>:"Set Unit ID.vi"("error in"=w757, "unit ID"=u8 2, "Modbus master in"=w756) -> ("error out"=w758:errorcluster, "Modbus master out"=w759:refnum<class "Modbus Master.lvclass">)  [unwired: 7 in]
        n290 = call "E700-Inverter Control.vi"("error in (no error)"=w758, "ON/OFF - Switch"=FALSE, "Modbus Master in"=w759) -> ("error out"=w763:errorcluster, "Modbus Master out"=w762:refnum<class "Modbus Master.lvclass">)  [unwired: 7 in]
        n291 = Bundle By Name(cluster=w764, "Rotation Instance"=w762) -> (w765:T4)
        n292 = call <vilib>:"Add State(s) to Queue__JKI_lib_State_Machine.vi"("State(s) in (\"\")"=w767) -> ("States Out"=w766:string)  [unwired: 14 in]
      }
    }
  }
